vi "AlliGator Image Actions.vi"(0 "AlliGator Q Elements":T6[](array[typedef]), 1 "VI in":refnum<vi>, 2 "Script in":bool, 5 "AlliGator IV DVR in":refnum<data-value>, 7 "AlliGator Q Event in":T7=enum."GUI:Idle", 9 "Data":variant, 11 "error in (no error)":errorcluster, 12 "AlliGator Ctrl Refnums":T8) -> (3 "Script out":bool, 4 "Alligator Queue Elements":T6[](array[typedef]), 6 "AlliGator IV DVR out":refnum<data-value>, 10 "[Notebook Message]":T1[](array[typedef]) {"Message Style"."Font Size" min=6.0 step=1.0}, 15 "error out":errorcluster)   [LabVIEW 2021, in "AlliGator Action Engine.lvlib"]
doc: "Processes AlliGator source image-related actions."
uses:
  AlliGator Action Engine.lvlib
  Internal Variables/AlliGator Internal Variables v2.ctl
  <vilib>/vision/Image Controls.llb/IMAQ Image.ctl
  Internal Variables/AlliGator Gate Image Set.ctl
  Files/AlliGator FLI Dataset Type.ctl
  Files/AlliGator Data Series Type.ctl
  Dual-Channel Datasets/AlliGator Dataset Channel.ctl
  Settings/AlliGator Gate Arithmetic.ctl
  Source Image/AlliGator Displayed Image.ctl
  Image/Named ROI Description.ctl
  Phasor Graph/AlliGator Decay Metadata v3.ctl
  Decay Analysis/Decay Preprocessing/AlliGator Decay Background Subtraction Info.ctl
  Decay Analysis/Decay Preprocessing/AlliGator Baseline Subtraction Method.ctl
  Graphs/XY Graph/XY Graph Plot Shift Parameters.ctl
  Graphs/XY Graph/XY Graph Plot Shift Method.ctl
  Decay Analysis/Decay Preprocessing/AlliGator Decay Extrapolation Parameters.ctl
  Phasor/Calibration Phasor (m, phi).ctl
  Phasor/Phasor Reference Series.ctl
  Phasor/Phasor Calibration Map v2.ctl
  Phasor/Phasor (g, s).ctl
  Phasor Graph/AlliGator Raw Phasor Plot Data v5.ctl
  Phasor/Phasor Standard Deviation Options.ctl
  Phasor Plot/AlliGator Phasor Multi-Harmonic Data.ctl
  Phasor/Phasor Harmonic Data.ctl
  Decay Fit Parameter Map/AlliGator Decay Fit Options & Parameters v4.ctl
  Fits/IRF(X)PSED/Decay Fit Options v4.ctl
  Fits/Decay Convolution/Decay Model.ctl
  Fits/Residual Type.ctl
  Fits/IRF(X)PSED/Fit Weights Type v2.ctl
  Fits/Non-linear Fitting Method v2.ctl
  Fits/Fit Calculation Method.ctl
  Fits/Non-linear Fitting Algorithm.ctl
  Decay Analysis/Decay Fit/AlliGator Decay Fit Parameter Constraints 2.ctl
  Fits/IRF(X)PSED/Decay Fit Parameters In List.ctl
  Fits/IRF(X)PSED/MLE Baseline Offset Type.ctl
  Decay Analysis/Decay Preprocessing/AlliGator Decay Preprocessing Parameters.ctl
  Fits/IRF(X)PSED/Decay Fit Parameters & Derived Quantities List v2.ctl
  Fits/IRF(X)PSED/Decay Fit Result Constraint.ctl
  Decay Fit Parameter Map/AlliGator Parameter Maps Data.ctl
  AlliGator Q Event.ctl
  GUI/AlliGator Ctrl Refnums.ctl
  GUI/AlliGator Other Ctrl Refnums.ctl
  GUI/AlliGator State Indicator.ctl
  GUI/AlliGator Main Window Tabs.ctl
  GUI/AlliGator Phasor Plot Ctrl Refnums.ctl
  GUI/AlliGator Phasor Graph Ctrl Refnums.ctl
  Phasor/Phasor Calibration Type.ctl
  GUI/AlliGator Dataset Ctrl Refnums.ctl
  GUI/AlliGator Registered Events Ctrl Refnums.ctl
  GUI/AlliGator Image Histogram Control Refnums.ctl
  Histograms/Linear Histogram Options.ctl
  Histograms/Histogram Bin Option.ctl
  Histograms/Histogram Bin Position.ctl
  Decay Fit Parameter Map/AlliGator Decay Fit Map Control Refnums.ctl
  Parameter Map/AlliGator Parameter Map Control Refnums.ctl
  AlliGator Q Element.ctl
  Notebook/Notebook Message Object.ctl
  Rich Text Box/Text Formatting.ctl
  Rich Text Box/Text Colors.ctl
  Rich Text Box/Text Style.ctl
  Rich Text Box/Text Alignment.ctl
  Alligator Elements Order in Action Stack.ctl
  Globals, Variables, Constants/AlliGator Variables List.ctl
  Palette/Image Palette Information.ctl
  Image/Image Display Palette Type.ctl
  Rich Text Box/Text Format List.ctl
  Image/Image Display to Clipboard Options.ctl
  Settings/AlliGator Settings List.ctl
  ROIs/AlliGator ROI Manager Actions.ctl
  Image/Image Control ROI Description.ctl
  Image/Image Save File Format.ctl
  Files/AlliGator Saved TIFF Image Type.ctl
  ROIs/AlliGator Selected ROI.ctl
  Image/Image Control Refnum.ctl
  Utilities/Read-Write.ctl
  5e39216f-2ed3-4ea3-88fe-69bdc2580e7f.vi
  Variant/Variant to Data/Variant to [String].vi
  Variant/Variant to Data/Variant to String.vi
  AlliGator Add Single Action to Stack.vi
  Variant/Variant to Data/Variant to Boolean.vi
  Variant/Variant to Data/Variant to DBL.vi
  ROIs/AlliGator Source Image ROI Storage [SGL] v3.vi
  AlliGator Add Action Array to Stack.vi
  Variant/Variant to Data/Variant to I32.vi
  <vilib>/Utility/error.llb/Error Cluster From Error Code.vi
  <vilib>/ErrorRing/Error Ring.xnode
  Image/Image.lvlib
  Variant/Variant to Data/Variant to Data.lvlib
  GUI/GUI.lvlib
  Files/AlliGator Files.lvlib
  Image Profile Window/AlliGator Image Profile Window.lvlib
  Source Image/AlliGator Source Image.lvlib
  Globals, Variables, Constants/AlliGator Globals, Variables & Constants.lvlib
  Palette/Palette.lvlib
  Settings/AlliGator Settings.lvlib
  ROIs/AlliGator ROIs.lvlib
  Notebook/AlliGator Notebook.lvlib
  Internal Variables/AlliGator Internal Variables.lvlib
  Python Plugins API/AlliGator Python Plugins.lvlib
  Phasor Calibration/AlliGator Phasor Calibration.lvlib
  Utilities/Utilities.lvlib
  GUI/AlliGator GUI.lvlib
  Notebook/Notebook.lvlib
  Phasor/Phasor.lvlib
  Decay Analysis/Decay Preprocessing/AlliGator Decay Preprocessing.lvlib
  Graphs/XY Graph/XY Graph Add-Ons.lvlib
  Phasor Graph/AlliGator Phasor Graph.lvlib
  Phasor Plot/AlliGator Phasor Plot.lvlib
  Fits/Fits.lvlib
  Decay Analysis/Decay Fit/AlliGator Decay Fit.lvlib
  Decay Fit Parameter Map/AlliGator Decay Fit Parameter Map.lvlib
  Rich Text Box/Rich Text Box.lvlib
  Dual-Channel Datasets/AlliGator Dual-Channel Datasets.lvlib
  Histograms/Histogram Window.lvlib
  Parameter Map/AlliGator Parameter Map.lvlib
panel:
  # "Drop the content of this VI on AlliGator's diagram\nIn AlliGator, replace the subVI template by a new version"
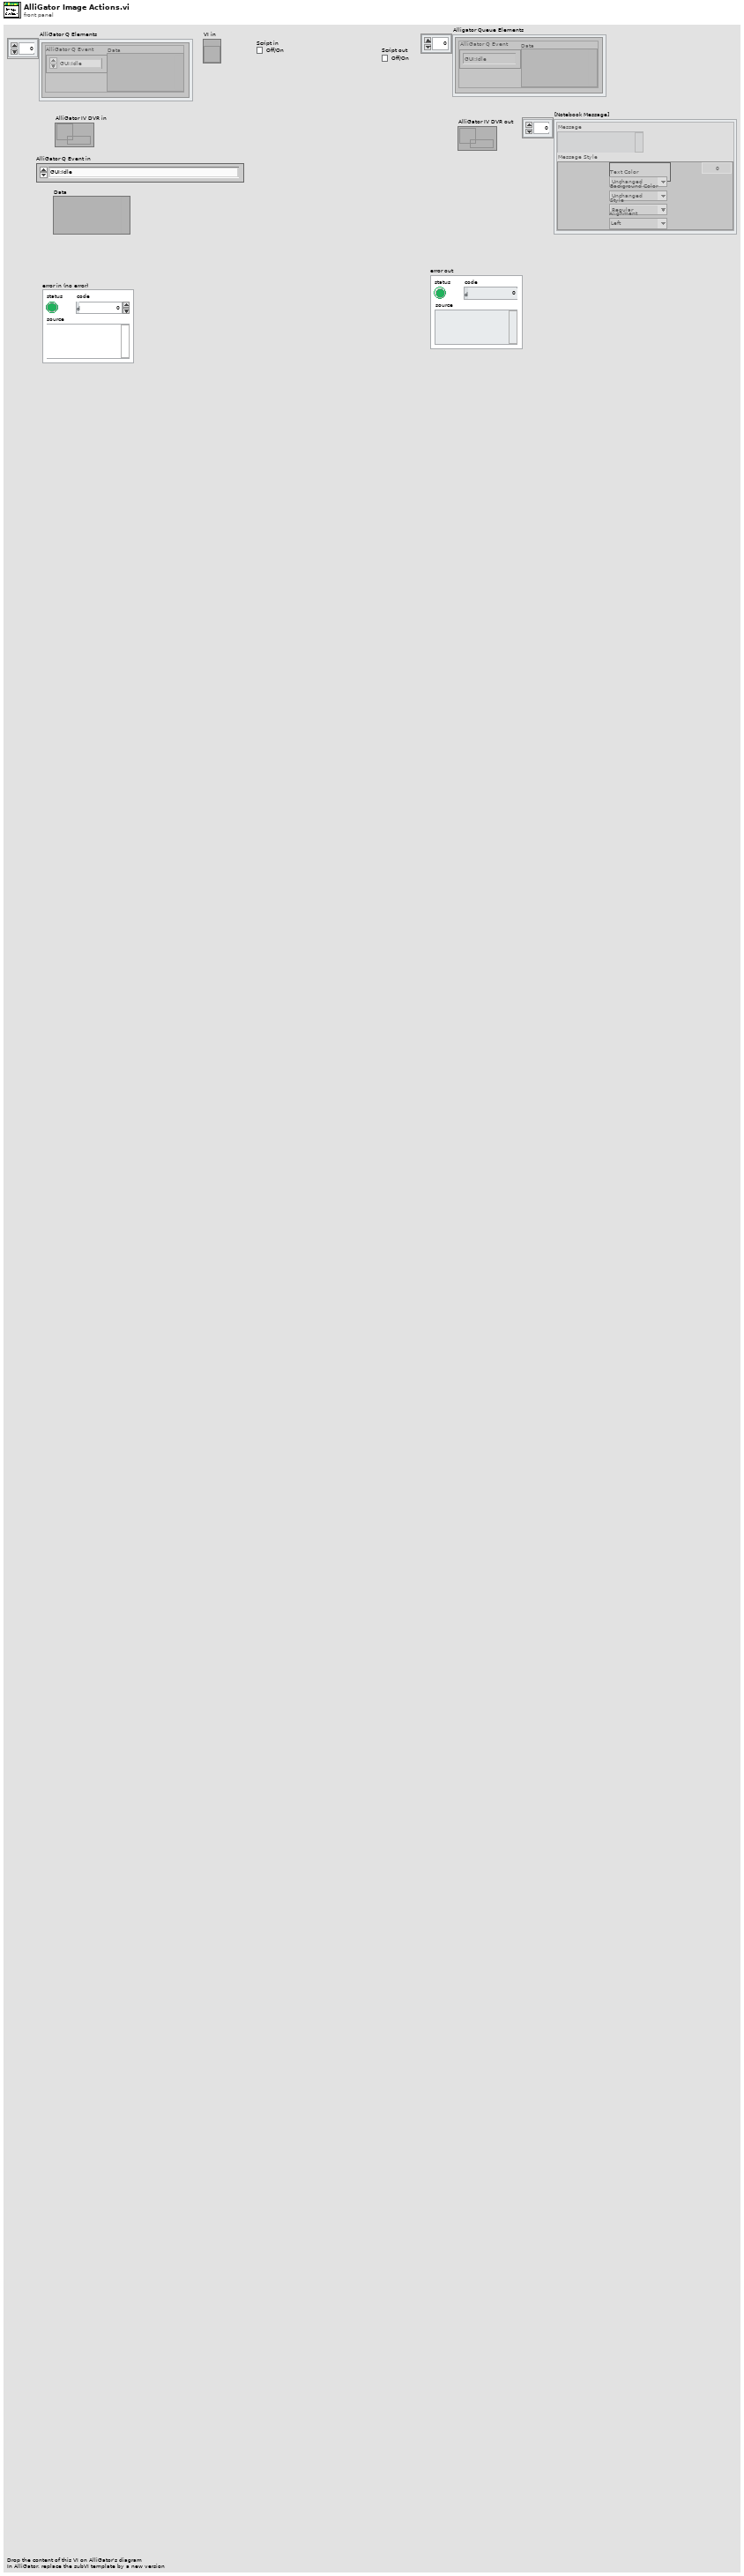
[diagram p1: front panel]
types:
  T1 = typedef "Notebook.lvlib/Notebook Message Object.ctl" = cluster{"Message":string, "Message Style":T2}
  T2 = typedef "Rich Text Box.lvlib/Text Formatting.ctl" = cluster{"Font":string, "Text Color":T3, "Background Color":T3, "Style":T4, "Font Size":dbl, "Alignment":T5}
  T3 = typedef "Rich Text Box.lvlib/Text Colors.ctl" = enum16{"Unchanged", "Black", "Blue", "Cyan", "Maroon", "Gray", "Violet", "Green", "Light Green", "Orange", "Yellow", "Magenta", "Red", "White"}
  T4 = typedef "Rich Text Box.lvlib/Text Style.ctl" = enum16{"Regular", "Bold", "Italic", "Underline", "Strikeout"}
  T5 = typedef "Rich Text Box.lvlib/Text Alignment.ctl" = enum16{"Left", "Right", "Center"}
  T6 = typedef "AlliGator Action Engine.lvlib/AlliGator Q Element.ctl" = cluster{"AlliGator Q Event":T7, "Data":variant}
  T7 = typedef "AlliGator Action Engine.lvlib/AlliGator Q Event.ctl" = enum16{"---- Files ----", "Files:Set Batch Export Files To Save", "Files:Set Dataset Loading & Pre-processing Options", "Files:Check #Frames in Dataset", "Files:Increment Frame Index", "Files:Open Mask Image", "Files:Open White Light Image", "Files:Open Single Dataset", "Files:New Folder of Folders Selected", "Files:Load File (all Types)_Scriptable", "Files:Move Flattened Series to Folders Series", "Files:Select Folder", "Files:Load FLI Dataset", "Files:Load Swiss SPAD 1 Dataset", "Files:Load Swiss SPAD 2 Dataset", "Files:Load .sdt FLI Dataset", "Files:Load .ptu FLI Dataset", "Files:Load .bin FLI Dataset", "Files:Load Single Gate Image Folder", "Files:Load I/m/phi Dataset (deprecated)", "Files:Load Single Image", "Files:Subtract Background File", "Files:Export FLI Dataset", "Files:Load HDF5 FLI Dataset", "Files:Set Destination File Path", "Files:Save Mask Image", "Files:Batch Conversion", "Files:New Folder Selected", "Files:Close FLI Dataset", "Files:Close FLI Dataset Series", "Files:Close White Light Image", "Files:Close Mask Image", "---- FLI Dataset ----", "FLI Dataset:Channel Arithmetic", "FLI Dataset:Export Average Lifetime Map as ASCII", "FLI Dataset:Export User-Defined Quantity Map as ASCII", "FLI Dataset:Python Function FLI Dataset Event", "FLI Dataset:ROI Analysis", "FLI Dataset:Tilted Logistic Square Gated IRF Characteristics Map", "FLI Dataset:Logistic Square Gated IRF Characteristics Map", "FLI Dataset:Square Gated IRF Characteristics Map", "FLI Dataset:Multi-ROI Single-Pixel Phasor Analysis", "FLI Dataset:Multi-ROI Single-Pixel NLSF Analysis", "FLI Dataset:All ROIs IRF Extraction", "FLI Dataset:All ROIs Decay Fit Non-Interactive (Fast + Individual IRF)", "FLI Dataset:All ROIs Phasor Analysis", "FLI Dataset:All ROIs Decay Fit", "FLI Dataset:Fluorescence Decay Statistics", "FLI Dataset:Update Decay Statistics Graph", "FLI Dataset:Get Decay from ROI", "FLI Dataset:All ROIs Average Lifetimes", "FLI Dataset:Save/Load Local IRFs", "FLI Dataset:Clear Local IRFs", "FLI Dataset:Phasor Calibration Maps (# Gates Series) Script", "FLI Dataset:Calibrated Phasor Map Series", "---- FLI Dataset Series ----", "FLI Dataset Series:Sum All Datasets in Series", "FLI Dataset Series:Add Dataset to Accumulated Dataset", "FLI Dataset Series:Display Accumulated Dataset", "FLI Dataset Series:Clear Dataset Series Sum", "FLI Dataset Series:Time-Series Analysis (NLSF)", "FLI Dataset Series:Time-Series Analysis (Phasor)", "---- Image ----", "Image:Update Image Profile Plots", "Image:Image Histogram Cursor Move", "Image:Image Histogram", "Image:Image Contrast", "Image:Set Image Histogram Cursor Move Flag", "Image:Clear Image Overlay", "Image:Use ROI as Search Area", "Image:Set ROI Diameter", "Image:Save Image Data as TIFF", "Image:Save Displayed Image with Overlay", "Image:Save Image Overlay Only", "Image:Save Image as Hot Pixel Mask", "Image:Change Source Image Color Palette", "Image:Copy Image to Clipboard", "Image:Source Image ROI Selection", "Image:Delete All ROIs", "Image:Delete All Unselected ROIs", "Image:Delete ROI", "Image:Merge All ROIs", "Image:Store ROI", "Image:Source Image ROI Storage", "Image:Export ROI Description to Notebook", "Image:Save ROI", "Image:Load ROI", "Image:Paste ROI Definition", "Image:Clear ROI", "Image:Identify ROIs in Mask Image", "Image:Create Complementary ROI", "Image:Create Contour ROI", "Image:Create ROI(s) from Pixels with Peak above Min_Scriptable", "Image:Create ROI(s) from Pixels with Intensity above Min_Scriptable", "Image:Compute ROI Statistics", "Image:Delete ROI(s) based on ROI Characteristics", "Image:Create ROI Grid", "Image:ROI to Individual Pixel ROIs", "Image:Python Function Source Image Event", "Image:Show Phasor Calibration Map ROI Centers", "Image:Convert ROI to Mask Image", "Image:Mouse Move", "Image:Mouse Up", "Image:Set Source Image Mouse Move Flag", "Image:Add Scale Bar Overlay", "Image:Delete Existing ROIs Option", "Image:Overlay ROI Median", "Image:Check Current ROI", "Image:Update True Pixel Value", "---- Decay ----", "Decay:Clear IRF/Reference Plot", "Decay:Add Decay to Graph", "Decay:Smoothen Plot", "Decay:Smoothen Plot Tail", "Decay:Average Selected Plots", "Decay:Extract IRF", "Decay:Optimal IRF Extraction", "Decay:Threshold IRF", "Decay:Fit to Model IRF", "Decay:Fit IRF to Square Gate", "Decay:Fit IRF to Logistic Square Gate", "Decay:Fit IRF to Tilted Logistic Square Gate", "Decay:Create Bounding Cursors Set", "Decay:Export Bounding Cursors Definition to Notebook", "Decay:Denoise Plot", "Decay:Compute Cumulative Function", "Decay:Use as Reference Decay", "Decay:Show Reference Decay/IRF", "Decay:Extrapolate Decay", "Decay:Create Head & Tail Bounding Cursors", "Decay:Store Cursor-defined Head & Tail Fractions", "Decay:Rebin Plot", "Decay:1-Normalize Decay", "Decay:[0-1]-Normalize Plot", "Decay:Straighten Decay", "Decay:Shift Decay", "Decay:Fold Decay", "Decay:Fit Decay", "Decay:Global Fit of Selected Decays", "Decay:Post Global Fit Script", "Decay:Add Global Fit Parameters to Graph", "Decay:Add Decay Parameter(s) to Plot (Graph)", "Decay:Export Decay to Phasor Graph", "Decay:Compute Average Lifetime", "Decay:Plot Convolution", "Decay:Graph Tip Strip Update", "---- Decay Statistics ----", "Decay Statistics:Tip Strip Update", "---- Intensity Time Trace ----", "Intensity Time Trace:Use File Timestamp", "Intensity Time Trace:Load Intensity Corrections File", "Intensity Time Trace:Clear Intensity Corrections File", "Intensity Time Trace:Tip Strip Update", "---- Phasor Plot ----", "Phasor Plot:Build Phasor Plot", "Phasor Plot:Change Phasor Plot Color Palette", "Phasor Plot:Adjust Phasor Plot Display Range", "Phasor Plot:Highlight Image ROI in Phasor Plot", "Phasor Plot:Save Phasor Plot Image with Overlay", "Phasor Plot:Export Complex Phasor Map", "Phasor Plot:Export Phasor Ratio Map", "Phasor Plot:Export Average Lifetime Map", "Phasor Plot:Compute Phase Lifetime Histogram", "Phasor Plot:Compute Phasor Ratio Histogram", "Phasor Plot:Compute Phase Lifetime vs Intensity Scatter Plot", "Phasor Plot:Weber 2-Component Decomposition", "Phasor Plot:Update Phasor Color Map Vertices", "Phasor Plot:Clear Phasor Overlay", "Phasor Plot:Use Segment Extremities as References", "Phasor Plot:Use UC/Segment Intersections as References", "Phasor Plot:Use UC/Principal Axis Intersections as References", "Phasor Plot:Use UC/Linear Fit Intersections as References", "Phasor Plot:Update Phasor Plot Reference", "Phasor Plot:Show Local Phasor Info in Phasor Plot", "Phasor Plot:Update Phasor Plot State", "Phasor Plot:Phasor Plot ROI Storage", "Phasor Plot:Phasor Plot ROI Selection", "Phasor Plot:Python Function Phasor Plot Event", "Phasor Plot:Overlay Phasor ROI, Ratio or Map in Source Image", "Phasor Plot:Compute Decay of Selected Phasors", "Phasor Plot:Phasor at Image Pixel", "Phasor Plot:Mouse Move", "Phasor Plot:Mouse Up", "Phasor Plot:Display Range Mouse Move", "Phasor Plot:Set Mouse Move Flag", "Phasor Plot:Update True Phasor Plot Value", "---- Phasor Graph ----", "Phasor Graph:Get Phasor Value", "Phasor Graph:Create New Phasor Plot Dialog", "Phasor Graph:Update Last Phasor Value", "Phasor Graph:Update Phasor (m, phi)", "Phasor Graph:Remove Single Phasor from Plot", "Phasor Graph:Add Single Phasor to Plot", "Phasor Graph:Remove Phasor Plot", "Phasor Graph:Remove Selected Phasor Plots", "Phasor Graph:Clear Phasor Data", "Phasor Graph:Clear Phasor Graph", "Phasor Graph:Cursor Move", "Phasor Graph:Draw Cursor Connecting Line", "Phasor Graph:Clear Cursor Connecting Line", "Phasor Graph:Find UC Intersection", "Phasor Graph:Use UC/Cursor-Defined Line Intersections", "Phasor Graph:Use Selected Plots Fitted Line/UC Intersections", "Phasor Graph:Use Selected Plots Principal Axis/UC Intersections", "Phasor Graph:Show Single Phasor", "Phasor Graph:Save Single Phasor Plot", "Phasor Graph:Save All Phasor Plots", "Phasor Graph:Load Phasor Plot(s)", "Phasor Graph:Phasor Multiplication", "Phasor Graph:Compute Average Phasor", "Phasor Graph:Compute Multiple Average Phasors (Selected Plots)", "Phasor Graph:Export Single Phasor Plot Phase Lifetimes", "Phasor Graph:Parameter 2 vs Parameter 1 Scatter Plot", "Phasor Graph:Use Cursor n Location", "Phasor Graph:Set Reference n to Current Phase Lifetime Value", "Phasor Graph:Set Reference n to Lifetime Value", "Phasor Graph:Set Cursor n Location", "Phasor Graph:Save Phasor Graph Image", "Phasor Graph:Update SEPL Plot", "Phasor Graph:Export Single Phasor Plot Data", "Phasor Graph:Export Selected Phasor Plots Data", "Phasor Graph:Python Function Phasor Graph Event", "Phasor Graph:Tip Strip Update", "---- Calibration ----", "Calibration:Set Calibration Type", "Calibration:Load/Save Phasor Calibration", "Calibration:Load/Save Phasor Calibration Series", "Calibration:Load/Save Phasor Calibration Map", "Calibration:Use as Calibration", "Calibration:Compute Optimal Calibration from Phasor References", "Calibration:Clear Phasor Calibration", "Calibration:Single Phasor Calibration Information", "Calibration:Use as Calibration Series", "Calibration:Use as Calibration Map", "Calibration:Clear Calibration Series", "Calibration:Phasor Calibration Series Information", "Calibration:Clear Calibration Map", "Calibration:Phasor Calibration Map Information", "Calibration:Apply Phasor Calibration", "Calibration:Update Single Plot Calibration", "Calibration:Update Multiple Plots Calibration", "Calibration:Clear Single Plot Calibration", "Calibration:Clear All Plots Calibrations", "Calibration:Clear Plot(s) Calibration(s)?", "---- Phasor Ratio ----", "Phasor Ratio:Clear Reference n", "Phasor Ratio:Toggle Selected Plot(s)  Lock to Reference 1", "Phasor Ratio:Use as Reference n", "Phasor Ratio:Send Reference n to Notebook", "Phasor Ratio:Toggle Selected Plot(s)  Lock to Reference 2", "Phasor Ratio:Compute Phasor Ratio at Mouse Location", "Phasor Ratio:Compute Phasor Plot's Average Phasor Ratio", "Phasor Ratio:Compute Time-Series Phasor Ratios", "Phasor Ratio:Fit Line to Phasor Ratio Plot", "Phasor Ratio:Save References", "Phasor Ratio:Load References", "Phasor Ratio:Update Phasor Reference 1", "Phasor Ratio:Update Phasor Reference 2", "Phasor Ratio:Move Cursor n to Reference n", "Phasor Ratio:Use as Phasor Reference 1 Lifetime", "Phasor Ratio:Use as Phasor Reference 2 Lifetime", "Phasor Ratio:Export Phasor Ratio Map as ASCII", "Phasor Ratio:Tip Strip Update", "---- Lifetime & Other Parameters Graph ----", "Lifetime:Compute Sliced Mean, SDV and CV Plots", "Lifetime:Plot Decay Shifts", "Lifetime:Plot Histogram", "---- Decay Fit Parameter Map ----", "Decay Fit Parameter Map:Export ROI NLSF Data as ASCII", "Decay Fit Parameter Map:Set Decay Fit Parameter Map Selection", "Decay Fit Parameter Map:Build Decay Fit Parameter Map", "Decay Fit Parameter Map:Change Decay Fit Parameter Map Color Palette", "Decay Fit Parameter Map:Export Decay Fit Parameter Map Data as ASCII", "Decay Fit Parameter Map:Export All Decay Fit Parameter Maps Data as ASCII", "Decay Fit Parameter Map:Selected Parameter Scatterplot", "Decay Fit Parameter Map:Parameter 2 vs Parameter 1 Scatterplot", "Decay Fit Parameter Map:Save Decay Fit Parameter Map Image", "Decay Fit Parameter Map:Save-Load IRFs & Fit Data", "Decay Fit Parameter Map:Update Local Decay Plots", "Decay Fit Parameter Map:Python Function Decay Fit Parameters Map Event", "Decay Fit Parameter Map:Overlay Decay Fit Parameter Map in Source Image", "Decay Fit Parameter Map:Selected Parameter vs Intensity Scatterplot", "Decay Fit Parameter Map:Mouse Up", "Decay Fit Parameter Map:Mouse Move", "Decay Fit Parameter Map:Display Range Mouse Move", "Decay Fit Parameter Map:Change Map Resolution", "Decay Fit Parameter Map:Variance Significance Maps", "Decay Fit Parameter Map:Fit Result Constraints Window", "---- Parameter Map ----", "Parameter Map:Export ROI Parameters Data as ASCII", "Parameter Map:Add Parameter Map Set", "Parameter Map:Delete Parameter Map Set", "Parameter Map:Update Parameter List", "Parameter Map:Build Parameter Map", "Parameter Map:Change Parameter Map Color Palette", "Parameter Map:Export Parameter Map Data as ASCII", "Parameter Map:Export All Parameter Maps Data as ASCII", "Parameter Map:Selected Parameter Scatterplot", "Parameter Map:Parameter 2 vs Parameter 1 Scatterplot", "Parameter Map:Selected Parameter vs Intensity Scatterplot", "Parameter Map:Save Parameter Map Image", "Parameter Map:Save-Load IRFs & Parameter Maps (TODO)", "Parameter Map:Set Parameter Map Selection", "Parameter Map:Python Function Parameter Map Event", "Parameter Map:Overlay Parameter Map in Source Image", "Parameter Map:Update Local Decay Plots", "Parameter Map:Mouse Up", "Parameter Map:Mouse Move", "Parameter Map:Display Range Mouse Move", "---- Generic Graph ----", "Generic Graph:Generic XY Graph Event", "Generic Graph:Python Function XY Graph Event", "Generic Graph:New Plot", "Generic Graph:Save Plot", "Generic Graph:XY Plot Histogram", "Generic Graph:Set XY Graph Plot Name", "Generic Graph:Set Last Cursor Style", "Generic Graph:Tip Strip Update", "---- GUI ----", "GUI:Start Script", "GUI:Type of Displayed Image Changed", "GUI:Gate Image Slide Changed", "GUI:Show Busy Icon", "GUI:Show Busy Icon & Abort Button", "GUI:Hide Busy Icon", "GUI:Hide Busy Icon & Abort Button", "GUI:Abort", "GUI:End Script", "GUI:Start Timing", "GUI:End Timing", "GUI:Set State Indicator", "GUI:Send Parameters JSON Strings to Clipboard", "GUI:Set Gate Step", "GUI:Idle", "GUI:Initialization", "GUI:Quit", "GUI:Increment Dataset Index", "GUI:Set Dataset Index to -1", "GUI:Time Series Slider Moved", "GUI:Time Series Slider Changed", "GUI:Toggle Playback or Loop", "GUI:Playback Script", "GUI:Set Phasor Frequency", "GUI:Open Window", "GUI:Start Test Script", "GUI:End Test Script", "GUI:Set Verbose Mode", "GUI:Set Verbose Settings Mode", "DEBUG"}
  T8 = typedef "AlliGator GUI.lvlib/AlliGator Ctrl Refnums.ctl" = cluster{"Other AlliGator Ctrl Refnums":T9, "Phasor Plot Ctrl Refnums":T10, "Phasor Graph Ctrl Refnums":T11, "Dataset Control Refnums":T12, "Registered Events Ctrl Refnums":T13, "Image Histogram Ctrl Refnums":T14, "Decay Fit Map Ctrl Refnums":T15, "Parameter Map Ctrl Refnums":T16}
  T9 = typedef "AlliGator GUI.lvlib/AlliGator Other Ctrl Refnums.ctl" = cluster{"State Indicators":refnum<vi>, " Progress Bar":refnum<vi>, "Decay Graph Active":refnum<vi>, "Decay Statistics Bin":refnum<vi>, "Time Step":refnum<vi>, "Use File Timestamp":refnum<vi>, "Tab Control":refnum<vi>, "CPU":refnum<vi>, "Abort Fit":refnum<vi>, "Dataset File/Folder Path":refnum<vi>, "Abort ROI Creation":refnum<vi>, "Event LED":refnum<vi>, "Dataset File/Folder Path 2":refnum<vi>, "Dataset File/Folder Path 3":refnum<vi>, "Dataset File/Folder Path 4":refnum<vi>, "Dataset File/Folder Path 5":refnum<vi>, "Dataset File/Folder Path 6":refnum<vi>, "Dataset File/Folder Path 7":refnum<vi>, "Dataset File/Folder Path 8":refnum<vi>, "Dataset File/Folder Path 9":refnum<vi>, "Dataset File/Folder Path 10":refnum<vi>, "Dataset File/Folder Path 11":refnum<vi>}
  T10 = typedef "AlliGator GUI.lvlib/AlliGator Phasor Plot Ctrl Refnums.ctl" = cluster{"Phasor Ratio":refnum<vi>, "Modulus Lifetime":refnum<vi>, "Phasor at cursor (m, phi)":refnum<vi>, "Phase Lifetime":refnum<vi>, "Phasor at cursor (g, s)":refnum<vi>, "Phasor Plor Average Lifetime":refnum<vi>, "Phasor Plot Active":refnum<vi>, "Save Phasor Plot":refnum<vi>, "Image Overlay Color":refnum<vi>, "Phasor Plot Color Scale":refnum<vi>, "Reference 1 Button":refnum<vi>, "Reference 2 Button":refnum<vi>, "True Phasor Plot Value":refnum<vi>}
  T11 = typedef "AlliGator GUI.lvlib/AlliGator Phasor Graph Ctrl Refnums.ctl" = cluster{"Phasor Ratio":refnum<vi>, "Modulus Lifetime":refnum<vi>, "Phasor at cursor (m, phi)":refnum<vi>, "Phase Lifetime":refnum<vi>, "Phasor at cursor (g, s)":refnum<vi>, "Phasor Graph Average Lifetime":refnum<vi>, "Phasor Graph Active":refnum<vi>, "Save Phasor Graph":refnum<vi>, "Phasor Frame Slide":refnum<vi>, "Single Step Phasor":refnum<vi>, "Calibration Type":refnum<vi>, "Show Line":refnum<vi>, "Phase Lifetime 1":refnum<vi>, "Phase Lifetime 2":refnum<vi>, "Phasor Graph Frequency":refnum<vi>, "Phasor Reference 1 Control":refnum<vi>, "Phasor Reference 2 Control":refnum<vi>, "Calibration Lifetime":refnum<vi>, "Phase Lifetime SDV":refnum<vi>, "Average Lifetime SDV":refnum<vi>, "Phasor Ratio SDV":refnum<vi>, "Modulus Lifetime SDV":refnum<vi>}
  T12 = typedef "AlliGator GUI.lvlib/AlliGator Dataset Ctrl Refnums.ctl" = cluster{"Current Data":refnum<vi>, "Gate Image Slide":refnum<vi>, "Time Point Slide":refnum<vi>, "Current Time Stamp":refnum<vi>, "Save Image":refnum<vi>, "Displayed Image":refnum<vi>, "Overlay Mode":refnum<vi>, "Phasor Overlay Color":refnum<vi>, "Image Color Scale":refnum<vi>, "Use ROI as Search Area":refnum<vi>, "Source Image ROI Color":refnum<vi>, "True Pixel Value":refnum<vi>}
  T13 = typedef "AlliGator GUI.lvlib/AlliGator Registered Events Ctrl Refnums.ctl" = cluster{"Time Point Slider":refnum<vi>, "Phasor Plot Display Range":refnum<vi>, "Decay Graph":refnum<vi>, "Decay Statistics Graph":refnum<vi>, "Intensity Time Trace":refnum<vi>, "Phasor Graph":refnum<vi>, "Phasor Ratio Graph":refnum<vi>, "Lifetime Graph":refnum<vi>, "Phasor Plot Display":refnum<vi>, "Source Image Display":refnum<vi>, "Decay Fit Parameter Map Display Range":refnum<vi>, "Decay Fit Parameter Map Display":refnum<vi>, "Parameter Map Display Range":refnum<vi>, "Parameter Map Display":refnum<vi>, "Phasor Plot Display Range":refnum<vi>}
  T14 = typedef "AlliGator GUI.lvlib/AlliGator Image Histogram Control Refnums.ctl" = cluster{"Image Histogram":refnum<vi>, "Image Histogram Options":refnum<vi>, "Image Histogram Active":refnum<vi>, "Image Histogram Upper Percentile":refnum<vi>, "Image Histogram Lower Percentile":refnum<vi>, "Auto-Adjust Contrast":refnum<vi>}
  T15 = typedef "AlliGator Decay Fit Parameter Map.lvlib/AlliGator Decay Fit Map Control Refnums.ctl" = cluster{"Decay Fit Parameter Map Color Scale":refnum<vi>, "Decay Fit Parameter":refnum<vi>, "Max Parameter":refnum<vi>, "Min Parameter":refnum<vi>, "Decay Fit Parameter Map Display":refnum<vi>, "Decay Fit Parameter Map Display Range":refnum<vi>, "Decay Parameter Map X":refnum<vi>, "Decay Parameter Map Y":refnum<vi>, "Decay Parameter Map Value":refnum<vi>}
  T16 = typedef "AlliGator Parameter Map.lvlib/AlliGator Parameter Map Control Refnums.ctl" = cluster{"Parameter Map Color Scale":refnum<vi>, "Map Parameter":refnum<vi>, "Max Parameter":refnum<vi>, "Min Parameter":refnum<vi>, "Parameter Map Display":refnum<vi>, "Parameter Map Display Range":refnum<vi>, "Parameter Map Set":refnum<vi>, "Parameter Map X":refnum<vi>, "Parameter Map Y":refnum<vi>, "Parameter Map Value":refnum<vi>}
  T17 = typedef "AlliGator Action Engine.lvlib/Alligator Elements Order in Action Stack.ctl" = enum16{"Enqueue 2 AFTER 1", "Enqueue 2 BEFORE 1"}
  T18 = typedef "AlliGator Globals, Variables & Constants.lvlib/AlliGator Variables List.ctl" = enum16{"---- GUI ----", "GUI:Initialization Status", "GUI:State Indicators Refnum", "GUI:Original AlliGator Menu Items", "GUI:Current Action Loop State", "GUI:Script in progress", "GUI:Playback", "GUI:Loop Playback", "GUI:Search ROI Used", "GUI:Search ROI", "Decay Graph Max Legend Size", "Intensity Graph Max Legend Size", "Decay Statistics Graph Max Legend Size", "Phasor Graph Max Legend Size", "Phasor Ratio Graph Max Legend Size", "Lifetime Graph Max Legend Size", "---- Files ----", "Files:Export Dataset Frames as Individual Files", "Files:Show Batch Export Help Balloons", "Files:Frames in Dataset", "Files:ptu File Frame Start Indices", "Files:Current Frame in Dataset", "Files:Current Frame Timestamp", "Files:Dataset Loaded", "Files:Dataset Metadata", "Files:Dataset Channel", "Files:Dataset Data Description", "Files:Background Dataset Metadata", "Files:Background Dataset Channel", "Files:Background Dataset Data Description", "Files:Background File Subtraction", "Files:Background File Path", "Files:Background File Pile-up Correction", "Files:Background File Pixel Well Capacity", "Files:Background File Scaling Factor", "Files:Current Dataset Load Settings", "Files:Dataset Path", "Files:ICCD-specific Information", "Files:Macrotime Gate Separation", "------ Python Plugins ------", "Python Plugins:Information", "Python Plugins:Python Session", "Python Plugins:Valid Python Session?", "---- Source Image ----", "Source Image:ROIs", "Source Image:Current ROI", "Source Image:ROI Event Refnum", "X_Source Image:Display Range", "X_Source Image:Palette Information", "X_Source Image:Type of Displayed Image", "X_Time Gate Slider", "Source Image:Palette List", "Source Image:Scale", "Source Image:ROI Overlay Color", "Source Image:Overlay to Erase", "Source Image:Is Displayed Image Accumulated", "Source Image:White Light Image Modified", "Source Image:Mask Image Modified", "---- Image Profile Window ----", "Image Profile:Window Event Refnum", "Image Profile:IntensityType", "Image Profile:Intensity Average Type", "Image Profile:Intensity-weighted SDV", "Image Profile:Box Profile Type", "Image Profile:Window Open", "Image Profile:Plotted Fit Parameter", "------ Phasor Graph -------", "Phasor Graph:Show Line", "---- Phasor Plot ---", "Phasor Plot:Parameters Changed", "Phasor Plot:FLI Dataset Modified since last Calculation", "Phasor Harmonics Data", "Selected Phasor Harmonics", "Phasor Harmonic Manager Event Refnum", "Phasor Plot:ROIs", "Phasor Plot:Current ROI", "Phasor Plot:ROI Event Refnum", "Phasor Plot:Image Reference Points", "Phasor Plot:Computed", "Phasor Plot:Palette Information", "Phasor Plot:Palette List", "Phasor Plot:Phasor Ratio Palette Information", "Phasor Plot:Phasor Ratio Palette List", "Phasor Plot:Image Scale", "Phasor Plot:Image Overlay to Erase", "Phasor Plot:Image Elements to Update", "Phasor Plot:Current Calculation Parameters", "Phasor Plot:Current Calibration Options", "Phasor Plot:Reset Cumulated Phasor Plot", "Phasor Plot:Reference 1", "Phasor Plot:Lifetime Reference 1", "Phasor Plot:Reference 1 Frequency", "Phasor Plot:Reference 2", "Phasor Plot:Lifetime Reference 2", "Phasor Plot:Reference 2 Frequency", "---- Decay Analysis ----", "Number of Selected Decays to Fit", "LS Fit Results", "LAR Fit Results", "BS Fit Results", "Last Decay Max - Min", "Best Fit Parameters", "Best Fit Parameter Names", "Actual Size X", "Actual Size Y", "Binning X", "Binning Y", "Actual # Gates", "Dataset Number", "Gates to...", "Gates Skipped", "Gates to keep", "Gate Step", "Gate Separation", "Reversed Gates", "Pile-up Correction", "Pixel Well Capacity", "Background Subtracted", "Background Subtraction Method", "Background Definition Range", "Background File (deprecated)", "Number of Dataset Accumulated", "Array of Accumulated Dataset Paths", "Do Averaged Datasets", "Destination File Path", "Process Plot Target", "Use 1/D as Phasor Frequency", "---- Decay Fit Parameter Map -----", "Decay Fit Parameter Map:Palette Information", "Decay Fit Parameter Map:Palette List", "Decay Fit Parameter Map:X Resolution", "Decay Fit Parameter Map:Y Resolution", "Decay Fit Parameter Map:Use Decay Fit Result Constraints", "Decay Fit Parameter Map:Decay Fit Result Constraints", "Decay Fit Parameter Map:Decay Fit Result Constraints Applied", "---- Parameter Map ----", "Parameter Map:Palette Information", "Parameter Map:Palette List", "------- Local Decay Window ---------", "Local Decay Graph Window:Event Refnum", "Local Decay Graph Window:Use normalized IRF for convolution", "----- Miscellaneous ----", "Misc:Skippable Dialog Windows Status"}
  T19 = typedef "Palette.lvlib/Image Palette Information.ctl" = cluster{"Palette Name [# Colors,int?,inv?]":string, "Palette Type":T20, "Palette Colors":u32[], "Interpolate?":bool}
  T20 = typedef "Image.lvlib/Image Display Palette Type.ctl" = u32
  T21 = typedef "Notebook.lvlib/Text Format List.ctl" = enum16{"Message", "Result", "Error", "Setting", "Verbose", "Warning"}
  T22 = typedef "Image.lvlib/Image Display to Clipboard Options.ctl" = cluster{"Include Overlay (T)":bool, "Image Only (T)":bool}
  T23 = cluster{"CtlRef":refnum<vi>, "Image to Clipboard Options":T22}
  T24 = typedef "AlliGator Settings.lvlib/AlliGator Settings List.ctl" = enum16{"GUI:Visible Settings Tab", "GUI:Last Run Version", "Source Image:Use Image Histogram for Contrast", "Source Image:Low Count Pixels Rejection Options", "Source Image:High Count Pixels Rejection Options", "Source Image:Use Image Brightness", "Source Image:Blend Overlay with Image Background", "Source Image:Use Fixed ROI Diameter", "Source Image:ROI Diameter", "Source Image:ROI Center Color", "Source Image:Peak Threshold", "Source Image:Intensity Threshold", "Source Image:Image Binning Options", "Source Image:Image Smoothing Options", "Source Image:Image Histogram Active", "Source Image:Invert Binary Mask", "Source Image:Hot Pixel Removal", "Source Image:Overlay Analyzed ROI Center", "Source Image:Auto-Adjust Contrast", "Source Image:Histogram Lower Percentile", "Source Image:Histogram Upper Percentile", "Source Image:Save Source Image", "Source Image:Scale Bar Options", "Source Image:Image Resolution (Pixel Size)", "Source Image:Flatfield Correction", "Source Image:Show Dead Left Columns Correction", "Source Image:Dead Left Columns Correction", "Source Image:Image Pre-Processing Operations Order", "Source Image:Overlay ROI Median", "Source Image:Median Overlay Color", "Data Information:Gate Width", "Data Information:Nanotime Gate Separation", "Data Information:Macrotime Gate Separation", "Data Information:Gate Step", "Data Information:# Gates", "Data Information:Gate Image Exposure", "Data Information:Gate Image Integration", "Data Information:Gates to Skip", "Data Information:Gates to Keep", "Data Information:Define Gates to", "Data Information:Channel Name", "Data Information:Available Channel Names", "Data Information:Channel Arithmetic", "Data Information:Background File Subtraction", "Data Information:Background File", "Data Information:Background Scaling Factor", "Data Information:Background Pile-up Correction", "Data Information:Background Pixel Well Capacity", "Data Information:Laser Period", "Data Information:SYNC Period", "Data Information:Pile-up Correction", "Data Information:Pixel Well Capacity", "Data Information:Dataset Scaling Factor", "Fluorescence Decay_Decay Pre-Processing:Reverse Gates", "Fluorescence Decay_Decay Pre-Processing:Verbose Decay Pre-Processing", "Fluorescence Decay_Decay Pre-Processing:Use Decay Pre-Processing", "Fluorescence Decay_Decay Pre-Processing:Background Subtraction", "Fluorescence Decay_Decay Pre-Processing:Background Definition Range", "Fluorescence Decay_Decay Pre-Processing:Baseline Subtraction Method", "Fluorescence Decay_Decay Pre-Processing:Decay Pre-Processing Operations Order", "Fluorescence Decay_Decay Pre-Processing:Smoothing Parameter", "Fluorescence Decay_Decay Pre-Processing:Shift Decay", "Fluorescence Decay_Decay Pre-Processing:Decay Shift Parameters", "Fluorescence Decay_Decay Pre-Processing:Fold Decay", "Fluorescence Decay_Decay Pre-Processing:# Folds", "Fluorescence Decay_Decay Pre-Processing:1-Normalize Decay", "Fluorescence Decay_Decay Pre-Processing:[0-1]-Normalize Decay", "Fluorescence Decay_Decay Pre-Processing:Smoothen Decay", "Fluorescence Decay_Decay Pre-Processing:Extrapolate Decay", "Fluorescence Decay_Decay Pre-Processing:Use Periodicity", "Fluorescence Decay_Decay Pre-Processing:Use Cursors", "Fluorescence Decay_Decay Pre-Processing:Tail Fraction", "Fluorescence Decay_Decay Pre-Processing:Head Fraction", "Fluorescence Decay_Decay Pre-Processing:Additional Points", "Fluorescence Decay_Decay Pre-Processing:Straighten Decay", "Fluorescence Decay_Decay Pre-Processing:Constant Background", "Fluorescence Decay_Decay Pre-Processing:Pixel-Normalize Decay", "Fluorescence Decay_Advanced Analysis:Extract IRF instead of Decay", "Fluorescence Decay_Advanced Analysis:IRF Extraction Options", "Fluorescence Decay_Advanced Analysis:IRF Optimization Options", "Fluorescence Decay_Advanced Analysis:Square Pulse Options", "Fluorescence Decay_Advanced Analysis:IRF Order", "Fluorescence Decay_Advanced Analysis:IRF Time Constants", "Fluorescence Decay_Advanced Analysis:Wavelet Analysis Options", "Fluorescence Decay_Advanced Analysis:Average Lifetime Options", "Fluorescence Decay_Fit Options:Fit Options", "Fluorescence Decay_Fit Options:Use Legacy Fitting Approach", "Fluorescence Decay_Fit Options:Use Data Information Laser Period", "Fluorescence Decay_Fit Parameters:Displayed Fit Parameters", "Fluorescence Decay_Fit Parameters:Fit Parameter Constraints", "Fluorescence Decay_Fit Parameters:Export Tabulated Results", "Fluorescence Decay_Fit Parameters:MLE Baseline Offset Type", "Fluorescence Decay_Fit Parameters:MLE Baseline Offset", "Fluorescence Decay_Fit Parameters:Guess Parameter Names", "Fluorescence Decay_Fit Parameters:Guess Parameter Values", "Fluorescence Decay_Fit Parameters:Guess Parameters Options", "Fluorescence Decay_Fit Parameters:Optimal Offset Selection Criterion", "Fluorescence Decay_Styles:Show Last Decay Only", "Fluorescence Decay_Styles:Decay Graph Color Array", "Fluorescence Decay:Decay Graph Active", "Fluorescence Decay Statistics:Min Peak Value", "Fluorescence Decay Statistics:Reject Low Decay Peak Pixels", "Fluorescence Decay Statistics:Reject High Decay Peak Pixels", "Fluorescence Decay Statistics:Max Peak Value", "Time Traces:Use File Timestamp", "Time Traces:Time Step", "Time Traces:Use Intensity Correction File", "Time Traces:Intensity Correction File", "Phasor Plot:Phasor Plot Smoothing Options", "Phasor Plot:Phasor Plot Size", "Phasor Plot:Phasor Plot Graphics Options", "Phasor Plot:Cumulative Phasor Plot", "Phasor Plot:Use Phasor Brightness", "Phasor Plot:Blend Overlay with Phasor Background", "Phasor Plot:Save Phasor Plot", "Phasor Plot:Show References", "Phasor Plot:Phasor Ratio Decay Range", "Phasor Plot:Exponential Fading", "Phasor Plot:Phasor Ratio Reference Colors", "Phasor Plot:Reference Radius", "Phasor Plot:Show Color Map Vertices", "Phasor Plot:Phasor Plot Active", "Phasor Plot:Phasor Ratio Color Map Type", "Phasor Plot:Phasor Ratio Color Map", "Phasor Plot:Phasor Ratio Display Range", "Phasor Plot:Selected Image ROI(s)", "Phasor Plot:All Image ROIs", "Phasor Plot:Selected Phasor Plot ROI(s)", "Phasor Plot:All Phasor Plot ROIs", "Phasor Plot:Phasor Ratio Color-Coded Quantity", "Phasor Plot:Store Phasor Harmonics", "Phasor Plot:Draw Reference Segment", "Phasor Plot:User-Defined Quantity", "Phasor Plot:Color Scale High Color", "Phasor Plot:Color Scale Low Color", "Phasor Plot:Intensity-weighted Phasor Plot", "Phasor Graph:Phasor Frequency", "Phasor Graph:Phasor Ratio Type", "Phasor Graph:Pixel-level Phasor Computation", "Phasor Graph:Save Phasor Graph", "Phasor Graph:Phasor Graph Active", "Phasor Graph:Phasor SDV Options", "Phasor Graph:Intensity-weighted Phasor Graph", "Phasor Graph:Define Shortest Lifetime as", "Phasor Calibration:Use Backup Calibration if needed", "Phasor Calibration:Backup Calibration Type", "Phasor Calibration:Calibration Type", "Phasor Calibration:Calibration Lifetime", "Phasor Calibration:Calibration Map Algorithm", "Single-Exponential Phasor Locus (SEPL):Gate Parameters", "Single-Exponential Phasor Locus (SEPL):User-defined Gate", "Single-Exponential Phasor Locus (SEPL):User-defined IRF", "Single-Exponential Phasor Locus (SEPL):Phasor Parameters", "Single-Exponential Phasor Locus (SEPL):Decay & IRF Parameters", "Single-Exponential Phasor Locus (SEPL):Display Parameters", "Lifetime Analysis:Decay Analysis Parameters", "Lifetime Analysis:Lifetime Map Active", "Plugins:Python Settings", "Miscellaneous:Verbose Mode", "Miscellaneous:Beep after Script", "Miscellaneous:Saved Image File Format", "Miscellaneous:Exported Gate Image Settings", "Miscellaneous:Include Loading in Timing", "Miscellaneous:Verbose Settings Mode", "Miscellaneous:Histogram Options", "Miscellaneous:Beep on Error", "Miscellaneous:# Logical Processors Used", "Miscellaneous:ROI Description Max Characters", "Miscellaneous:Verbose Error Mode", "Miscellaneous:Transparent Mask Color"}
  T25 = typedef "AlliGator ROIs.lvlib/AlliGator ROI Manager Actions.ctl" = enum16{"Undefined", "Delete Current ROI", "Delete All Unselected ROIs", "Delete Multiple ROIs", "Delete All ROIs", "Swap ROIs", "Insert ROI", "Update Current ROI Descriptor", "Rename Current ROI", "Store New ROI", "Store Multiple ROIs", "Select Next ROI", "Select Previous ROI", "Find Selected ROI", "Show All ROIs", "Update ROI Manager Window", "Merge All ROIs", "Unmerge ROI", "Set Selected ROI by ID"}
  T26 = typedef "ROI Descriptor" = cluster{"Global Rectangle":i32[], "Contours":cluster{"ID":enum32{"External", "Internal"}, "Type":u32, "Coordinates":i32[]}[]}
  T27 = typedef "Image.lvlib/Image Control ROI Description.ctl" = cluster{"Image Control Label":string, "ROI Descriptor":T26}
  T28 = typedef "IMAQ Image.ctl" = refnum<image>
  T29 = typedef "Image.lvlib/Image Save File Format.ctl" = enum16{"PNG", "JPEG", "BMP"}
  T30 = typedef "AlliGator Files.lvlib/AlliGator Saved TIFF Image Type.ctl" = enum16{"Single Gate", "Sum of All Gates", "Phasor"}
  T31 = typedef "AlliGator ROIs.lvlib/AlliGator Selected ROI.ctl" = cluster{"Image Ctrl Ref":T32, "All ROIs?":bool}
  T32 = typedef "Image.lvlib/Image Control Refnum.ctl" = refnum<vi>
  T33 = typedef "Utilities.lvlib/Read-Write.ctl" = enum16{"Read", "Write"}
  T34 = typedef "AlliGator Internal Variables.lvlib/AlliGator Internal Variables v2.ctl" = cluster{"----------------------------- Images -----------------------------":u8, "Displayed Image":T28, "White Light Image":T28, "Mask Image":T28, "ROI Mask Image":T28, "Current Dataset Images 1":T35, "Background Dataset Images 1":T35, "Current Dataset Images 2":T35, "Background Dataset Images 2":T35, "Current Dataset Arithmetic Images":T35, "Accumulated Dataset Images 1":T35, "Accumulated Dataset Images 2":T35, "Accumulated Dataset Arithmetic Images":T35, "----------------------------- File Paths -----------------------------":u8, "Phasor Plot Image":T28, "Decay Fit Parameter Map Image":T28, "Parameter Map Image":T28, "Single Data Point Path":path, "White Light Image Path":path, "Mask Image Path":path, "Time-Series Folder":path, "[Time-Series Paths]":path[], "----------------------------- FLI Dataset -----------------------------":u8, "Current Dataset":i32, "Single Dataset Type":T36, "Current Folder":string, "AlliGator Data Series Type":T37, "# Datasets":i32, "Dual-Channel Dataset":bool, "Selected Channel Name":string, "Dataset Channel":T38, "Channel Arithmetic":T39, "Dual-Channel Background Dataset":bool, "Background Channel":T38, "Dual-Channel Accumulated Dataset":bool, "Start Time":dbl, "[Time-Series Timestamps]":dbl[], "[Intensity Corrections]":dbl[], "Time Series Script":bool, "Type of Displayed Image":T40, "Gate Image Slide":u16, "# Gates":i32, "ROIs":T41[], "----------------------------- Decays -----------------------------":u8, "ROI Decay":cluster{"t Array":dbl[], "I Array":dbl[]}, "Valid Decay":bool, "Decay  Metadata":T42, "Reference Decay Plot Name":string, "Reference Decay":cluster{"t Array":dbl[], "I Array":dbl[]}, "Decay Shift Plot":cluster{"Time Stamps":dbl[], "Decay Shifts":dbl[]}, "[Decays Max Values]":sgl[], "[Decays Min Values]":sgl[], "----------------------------- Calibration -----------------------------":u8, "Calibration Phasor":T48, "Calibration Phasor Series":T49, "Phasor Calibration Map":T50, "Calibration Map MD5 Digest":string, "----------------------------- Phasor Graph -----------------------------":u8, "Last Raw Phasor":T51, "Last Calibrated Phasor":T51, "Last Calibrated Phasor SDV":T51, "Phasor Graph:Phasor Plot":cluster{"g Array":dbl[], "s Array":dbl[]}, "Phasor Graph:Phasor SDV Plot":cluster{"g Array":dbl[], "s Array":dbl[]}, "[Phasor Graph:Raw Phasor Plots]":T52[], "Phasor Plot locked to Ref 1":i32, "[Phasor Plot(s) locked to Ref 1]":i32[], "[Phasor Plot(s) locked to Ref 2]":i32[], "[Pixel Phasors]":T51[], "----------------------------- Phasor Plot -----------------------------":u8, "[[Sum Image]]":dbl[][], "[[CSG Phasors]]":csg[][], "[[Valid Pixel?]]":bool[][], "[[Phasor Ratios]]":dbl[][], "[[Average Lifetimes]]":dbl[][], "Amplitude Weighted Average Lifetime":bool, "I/m/phi Dataset":cluster{"I/m/phi Dataset?":bool, "Base Frequency":dbl[unit], "Harmonic Orders":u8[]}, "Multi Phasor Plot Data":T54, "----------------------------- Decay Fit Parameter Map -----------------------------":u8, "Decay Fit Options & Parameters":T56, "Fit Options: Decay Preprocessing Parameters":T67, "Fit Options: Reference Decay":cluster{"t Array":dbl[], "I Array":dbl[]}, "Is Full Image Parameters Map":bool, "Is Single-Pixels Parameters Map":bool, "NLSF Parameters Map X Resolution":i32, "NLSF Parameters Map Y Resolution":i32, "[Single Decay Fit Parameters]":dbl[], "Fit Model":T58, "[[Multiple Decays Fit Parameters]]":dbl[][], "[[Multiple Decays Fit Parameter SDVs]]":dbl[][], "[[IRFs]]":dbl[][], "[ROI Descriptors]":T26[], "IRF Array Time Axis":dbl[], "Decay Array Time Axis":dbl[], "[Decay Fit Parameter Names]":T68[], "[Decay Sum]":dbl[], "Array of Decay Fit Result Constraints":T69[], "Selected ROIs Array":bool[], "----------------------------- Parameter Maps -----------------------------":u8, "[Map Set Names]":string[], "[Parameter Maps]":T70[], "[[User-defined Quantities]]":dbl[][], "User-defined Quantity":string}
  T35 = typedef "AlliGator Internal Variables.lvlib/AlliGator Gate Image Set.ctl" = cluster{"SGL Gate Images":T28[], "SGL Sum Image":T28, "SGL Max Image":T28, "SGL Min Image":T28}
  T36 = typedef "AlliGator Files.lvlib/AlliGator FLI Dataset Type.ctl" = enum16{"HDF5 FLI Dataset", "Gate Image Folder", ".sdt FLI Dataset (Becker & Hickl)", ".ptu FLI Dataset (PicoQuant)", "SS1 FLI Dataset", "SS2 FLI Dataset", "I/m/phi Dataset", ".bin FLI Dataset (PicoQuant Binned)", ".bin FLI Dataset (Piccolo Binned)", ".mat FLI Dataset"}
  T37 = typedef "AlliGator Files.lvlib/AlliGator Data Series Type.ctl" = enum16{"Not a Supported Series", "Gate Images Folder Series", "SwissSPAD 2 Dataset Series", "B&H FLI Dataset Series", "PicoQuant PTU FLI Dataset Series", "PicoQuant BIN FLI Dataset Series", "Piccolo hist BIN FLI Dataset Series", "HDF5 FLI Dataset Series"}
  T38 = typedef "AlliGator Dual-Channel Datasets.lvlib/AlliGator Dataset Channel.ctl" = enum16{"G2", "INT"}
  T39 = typedef "AlliGator Settings.lvlib/AlliGator Gate Arithmetic.ctl" = enum16{"None", "INT-G2", "G2/INT*<INT>", "(1 - G2/INT)*<INT>"}
  T40 = typedef "AlliGator Source Image.lvlib/AlliGator Displayed Image.ctl" = enum16{"Single Gate", "Sum of All Gates", "Max of All Gates", "Min of All Gates", "-", "White Ligth Image", "Mask Image"}
  T41 = typedef "Image.lvlib/Named ROI Description.ctl" = cluster{"ROI Descriptor":T26, "ROI Name":string, "Overlay Color":u32}
  T42 = typedef "AlliGator Phasor Graph.lvlib/AlliGator Decay Metadata v3.ctl" = cluster{"ROI Descriptor":T26, "ROI Center":cluster{"X":i32, "Y":i32}, "Decay Background Subtraction Info":T43, "Decay Reverted":bool, "Decay Smoothened":bool, "Decay Straightened":bool, "Fitted Tau (Decay Straightening)":dbl, "Decay Shift Parameters":T45, "Decay Shifted":bool, "Decay Extrapolated":bool, "Decay Extrapolation Parameters":T47, "Decay Normalized":bool, "Fold Decay":bool, "# Folds":u32}
  T43 = typedef "AlliGator Decay Preprocessing.lvlib/AlliGator Decay Background Subtraction Info.ctl" = cluster{"Laser Period":dbl[unit], "Gate Duration":dbl[unit], "Baseline Subtraction Method":T44, "Background Definition Range":cluster{"Min Gate":dbl[unit], "Max Gate":dbl[unit]}, "Total Intensity w/o Bkgd Subtraction":dbl, "Bkgd-subtracted Intensity (exp)":dbl, "# Data Points":i32, "Background/Gate":dbl, "Fitted Lifetime":dbl[unit], "Bkgd-subtracted Intensity (theo)":dbl}
  T44 = typedef "AlliGator Decay Preprocessing.lvlib/AlliGator Baseline Subtraction Method.ctl" = enum16{"Mean", "Min", "Square Gated Single-Exponential", "File", "Constant"}
  T45 = typedef "XY Graph Add-Ons.lvlib/XY Graph Plot Shift Parameters.ctl" = cluster{"Type":T46, "Shift":dbl[unit], "Threshold":dbl, "Rotate":bool}
  T46 = typedef "XY Graph Add-Ons.lvlib/XY Graph Plot Shift Method.ctl" = enum16{"Default", "CFD", "Threshold", "Cross-Correlation"}
  T47 = typedef "AlliGator Decay Preprocessing.lvlib/AlliGator Decay Extrapolation Parameters.ctl" = cluster{"Additional Points":u32, "Head Fraction":dbl, "Fitted Tau":dbl, "Use Periodicity":bool, "Use Cursors":bool, "Tail Fraction":dbl}
  T48 = typedef "Phasor.lvlib/Calibration Phasor (m, phi).ctl" = cluster{"m":dbl, "phi":dbl, "Phasor Frequency":dbl[unit], "Reference Lifetime":dbl[unit]}
  T49 = typedef "Phasor.lvlib/Phasor Reference Series.ctl" = cluster{"m Array":dbl[], "phi Array":dbl[], "Phasor Frequency":dbl[unit], "Calibration Lifetime":dbl[unit]}
  T50 = typedef "Phasor.lvlib/Phasor Calibration Map v2.ctl" = cluster{"Phasor Frequency":dbl[unit], "Calibration Lifetime":dbl[unit], "ROI Centers":cluster{"X":i32, "Y":i32}[], "ROI Descriptors":T26[], "Map Resolution X":i32, "Map Resolution Y":i32, "z Array":cdb[]}
  T51 = typedef "Phasor.lvlib/Phasor (g, s).ctl" = cluster{"g":dbl, "s":dbl}
  T52 = typedef "AlliGator Phasor Graph.lvlib/AlliGator Raw Phasor Plot Data v5.ctl" = cluster{"Phasor Plot Name":string, "Raw Phasor Plot":T51[], "Phasor Frequency":dbl[unit], "[Decay Metadata]":T42[], "Raw Phasor Plot SDV":T51[], "Phasor SDV Options":T53, "[Calibration Phasor]":T48[], "Intensity Array":dbl[]}
  T53 = typedef "Phasor.lvlib/Phasor Standard Deviation Options.ctl" = cluster{"Compute Estimated SDV":bool, "# Replicas":u32, "Use Estimated Average Phasor":bool}
  T54 = typedef "AlliGator Phasor Plot.lvlib/AlliGator Phasor Multi-Harmonic Data.ctl" = cluster{"Base Frequency":dbl[unit], "# Harmonics":u8, "Harmonic Orders":u8[], "Phasor Plot Settings Checksum":u64, "Phasor Harmonic Data Array":T55[]}
  T55 = typedef "Phasor.lvlib/Phasor Harmonic Data.ctl" = cluster{"Phasor Harmonic Name":string, "Phasor Plot Settings Checksum":u64, "Phasor Frequency":dbl[unit], "Base Frequency":dbl[unit], "Harmonic Order":u8, "Phasor Plot Parameters":string, "Phasor Array [[CSG]]":csg[][], "Dataset File Path":path}
  T56 = typedef "AlliGator Decay Fit Parameter Map.lvlib/AlliGator Decay Fit Options & Parameters v4.ctl" = cluster{"SYNC Period":dbl[unit], "Fit Options":T57, "Fit Parameter Constraints":T64[], "MLE Baseline Offset":dbl, "MLE Baseline Offset Type":T66}
  T57 = typedef "Fits.lvlib/Decay Fit Options v4.ctl" = cluster{"Show Fit Residuals":bool, "Fit Model":T58, "Residual Type":T59, "Max Decay Percentile":dbl, "Min Decay Percentile":dbl, "Show Full Decay":bool, "Weights":T60, "Fitting Method":T61, "Compute Parameter Uncertainties":bool, "Periodic Boundaries":bool, "Model Calculation":T62, "Period":dbl[unit], "Termination Criteria":cluster{"Max Iterations":i32, "Max Function Calls":i32, "Max Time":dbl[unit], "Function Tolerance":dbl, "Parameter Tolerance":dbl, "Gradient Tolerance":dbl, "Min Lambda":dbl, "Max Lambda":dbl, "Initial Tick Count":u32}, "Offset Resolution":dbl[unit], "Use Local IRF":bool, "Fitting Algorithm":T63, "Show Confidence Interval ":bool, "Confidence Level":dbl}
  T58 = typedef "Fits.lvlib/Decay Model.ctl" = enum16{"1-Exponential", "2-Exponentials"}
  T59 = typedef "Fits.lvlib/Residual Type.ctl" = enum16{"Standard", "Normalized", "Reduced"}
  T60 = typedef "Fits.lvlib/Fit Weights Type v2.ctl" = enum16{"Unweighted", "1/Variance (Neyman)", "1/Variance (Pearson)", "Best of All"}
  T61 = typedef "Fits.lvlib/Non-linear Fitting Method v2.ctl" = enum16{"Least Square", "Least Absolute Residual", "Bisquare", "MLE", "-", "Best of All"}
  T62 = typedef "Fits.lvlib/Fit Calculation Method.ctl" = enum16{"Simulation", "Convolution", "Integration"}
  T63 = typedef "Fits.lvlib/Non-linear Fitting Algorithm.ctl" = enum16{"Levenberg-Marquardt", "Trust-Region Dogleg"}
  T64 = typedef "AlliGator Decay Fit.lvlib/AlliGator Decay Fit Parameter Constraints 2.ctl" = cluster{"Fit Parameter":T65, "Min Value":dbl, "Max Value":dbl, "Global":bool, "Used":bool}
  T65 = typedef "Fits.lvlib/Decay Fit Parameters In List.ctl" = enum16{"Offset", "Baseline", "A_1", "tau_1", "A_2", "tau_2"}
  T66 = typedef "Fits.lvlib/MLE Baseline Offset Type.ctl" = enum32{"Absolute", "Percentage"}
  T67 = typedef "AlliGator Decay Preprocessing.lvlib/AlliGator Decay Preprocessing Parameters.ctl" = cluster{"Background Subtraction":bool, "Straighten Decay":bool, "Reverse Gates":bool, "1-Normalized Decay":bool, "Smoothen Decay":bool, "Smoothing Parameter":dbl, "Shift Decay":bool, "Decay Shift Parameters":T45, "Extrapolate Decay":bool, "Additional Points":u32, "Head Fraction":dbl, "Pixel-Normalize Decay":bool, "Use Periodicity":bool, "Use Cursors":bool, "Tail Fraction":dbl, "Use Decay Pre-Processing":bool, "Fold Decay":bool, "# Folds":u32, "[0-1]-Normalized Decay":bool}
  T68 = typedef "Fits.lvlib/Decay Fit Parameters & Derived Quantities List v2.ctl" = enum16{"Offset", "Baseline", "A_1", "tau_1", "A_2", "tau_2", "<tau>_a", "f1_a", "f2_a", "<tau>_i", "f1_i", "f2_i", "-", "R^2", "Chi^2"}
  T69 = typedef "Fits.lvlib/Decay Fit Result Constraint.ctl" = cluster{"Fit Parameter":enum16{"Offset", "Baseline", "A_1", "tau_1", "A_2", "tau_2", "<tau>_a", "f1_a", "f2_a", "<tau>_i", "f1_i", "f2_i", "-", "R^2", "Chi^2", "Max Relative Residual", "<Residual ACF>", "Residual ACF SDV", "tau_2/tau_1"}, "Min Value":dbl, "Max Value":dbl, "Use Constraint":bool}
  T70 = typedef "AlliGator Decay Fit Parameter Map.lvlib/AlliGator Parameter Maps Data.ctl" = cluster{"Map Set Name":string, "[Parameter Names]":string[], "[[Parameters]]":dbl[][], "[[Parameter SDVs]]":dbl[][], "Decay Array Time Axis":dbl[], "[[IRFs]]":dbl[][], "IRF Array Time Axis":dbl[], "X Resolution":i32, "Y Resolution":i32, "Intensity Array":dbl[]}
  T71 = typedef "Image.lvlib/Image ROI Statistics Selection.ctl" = cluster{"Area (pixels)":bool, "% of Image":bool, "Total Intensity":bool, "Mean Intensity":bool, "Median Intensity":bool, "Mode Intensity":bool, "Intensity Standard Deviation":bool, "Min Intensity":bool, "Max Intensity":bool, "Mean SNR":bool, "Median SNR":bool, "Mode SNR":bool, "SNR Standard Deviation":bool, "Max SNR":bool, "Min SNR":bool, "# Rejected Pixels (NaN, Inf)":bool, "# Negative Pixels":bool, "Long Axis Length":bool, "Short Axis Length":bool, "Aspect Ratio":bool}
  T72 = cluster{"Global Rectangle":i32[], "Contours":cluster{"Contour Type":u32, "ROI Type":u32, "Points":i32[]}[]}
  T73 = typedef "Image.lvlib/Image Control ROI Description v2.ctl" = cluster{"Image Control Label":string, "Named ROI Description":T41}
  T74 = typedef "Image.lvlib/Image Display User Event Data.ctl" = cluster{"Image Control Refnum":T32, "Coords":T75, "button info":cluster{"button 1":bool, "button 2":bool, "button 3":bool, "button 4":bool}, "keys pressed":enum16{"0", "1", "2", "3", "4", "5", "6", "7", "8", "9", "A", "B", "C", "D", "E", "F", "G", "H", "I", "J", "K", "L", "M", "N", "O", "P", "Q", "R", "S", "T", "U", "V", "W", "X", "Y", "Z", "F1", "F2", "F3", "F4", "F5", "F6", "F7", "F8", "F9", "F10", "F11", "F12", "F13", "F14", "F15", "ADD", "BACK", "BACKSLASH", "CAPITAL", "COMMA", "DECIMAL", "DELETE", "DIVIDE", "DOWN", "END", "EQUALS", "ESCAPE", "GRAVE (`)", "HOME", "INSERT", "LBRACKET", "LCONTROL", "LEFT", "L ALT", "LSHIFT", "LWIN", "MINUS", "MULTIPLY", "NEXT", "NUMLOCK", "NUMPAD_0", "NUMPAD_1", "NUMPAD_2", "NUMPAD_3", "NUMPAD_4", "NUMPAD_5", "NUMPAD_6", "NUMPAD_7", "NUMPAD_8", "NUMPAD_9", "PAUSE", "PERIOD", "PRIOR (PG UP)", "RBRACKET", "RCONTROL", "RETURN", "RIGHT", "R ALT", "RSHIFT", "RWIN", "SCROLL", "SEMICOLON", "SLASH", "SPACE", "SUBTRACT", "TAB", "UP", "ENTER (num pad)", "' (quote)"}[]}
  T75 = typedef "LVPoint32TypeDef.ctl" = cluster{"Horizontal":i32, "Vertical":i32}
  T76 = typedef "AlliGator GUI.lvlib/AlliGator Image Mouse Up Event Data.ctl" = cluster{"Current ROI Tool":u32, "ROI Descriptor":T77, "Shift":bool, "Alt":bool, "Image Display Refnum":T32}
  T77 = typedef "Image.lvlib/Image ROI Descriptor.ctl" = cluster{"Global Rectangle":i32[], "Contours":T78[]}
  T78 = typedef "Image.lvlib/Image Contour Definition.ctl" = cluster{"Contour Type":T79, "ROI Type":T80, "Points":i32[]}
  T79 = typedef "Image.lvlib/Image Contour ID.ctl" = enum32{"External", "Internal"}
  T80 = typedef "Image.lvlib/Image ROI Type.ctl" = enum16{"No Selection", "Point", "Line", "Rectangle", "Oval", "Polygon", "Freehand Region", "Annulus", "Unused2", "Unused3", "Broken Line", "Freehand Line", "Rotated Rectangle"}
  T81 = typedef "Image.lvlib/Image Display Event.ctl" = cluster{"Item Tag":string, "Image Control Refnum":T32, "Coords":T75, "Item Path":string}
  T82 = typedef "AlliGator ROIs.lvlib/AlliGator ROI Selection Data.ctl" = cluster{"Action":T25, "ID":i32}
  T83 = typedef "Fits.lvlib/Decay Fit Parameters & Derived Quantities List.ctl" = enum16{"Offset", "Baseline", "A_1", "tau_1", "A_2", "tau_2", "<tau>_a", "f1_a", "f2_a", "<tau>_i", "f1_i", "f2_i", "-", "R^2", "Chi^2"}
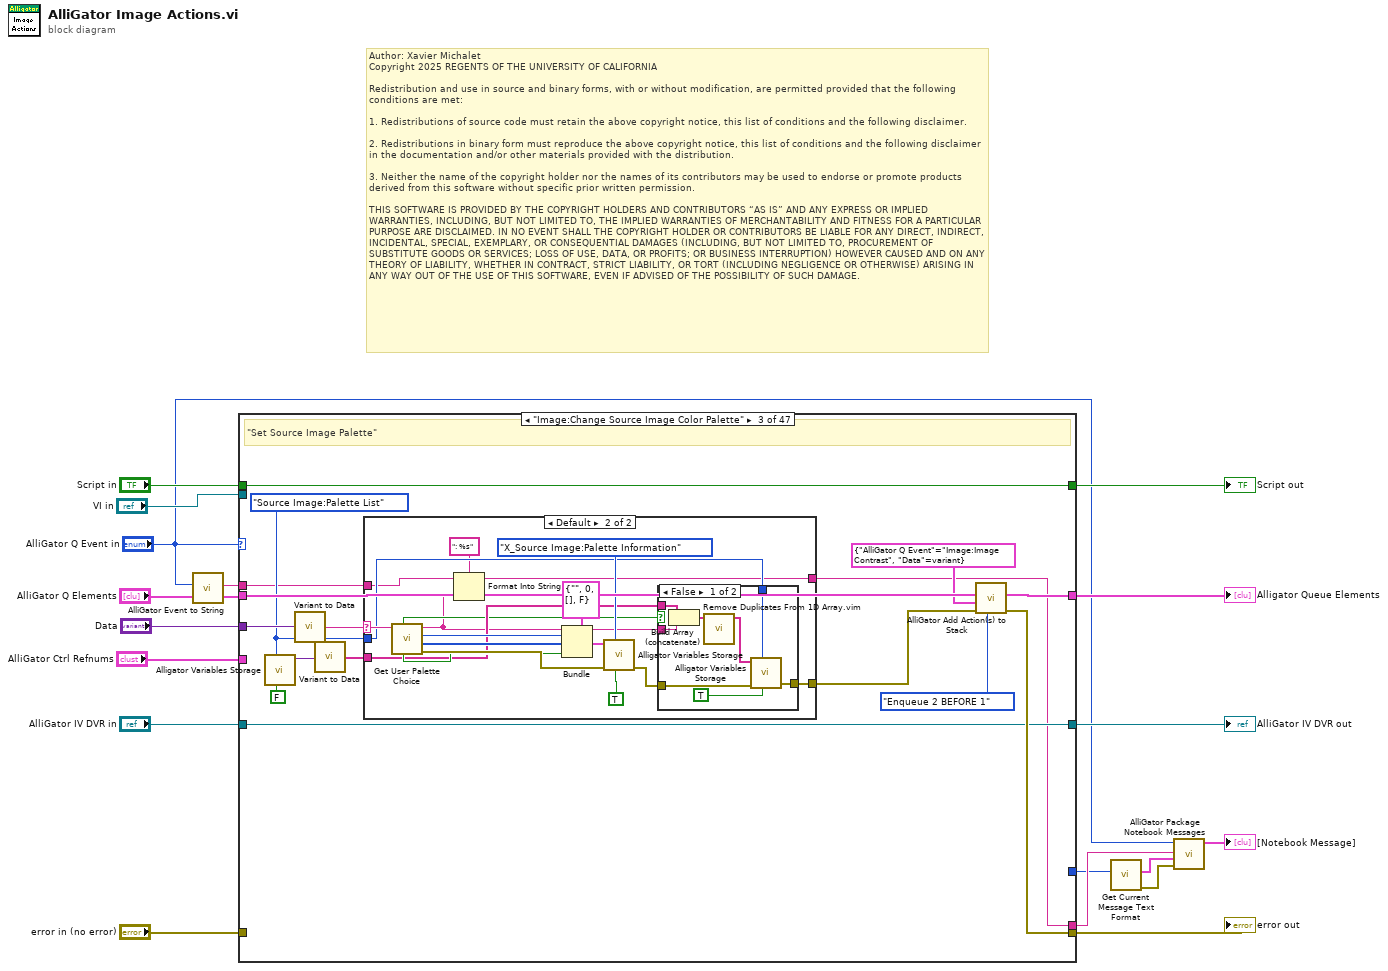
[diagram p0: block diagram]
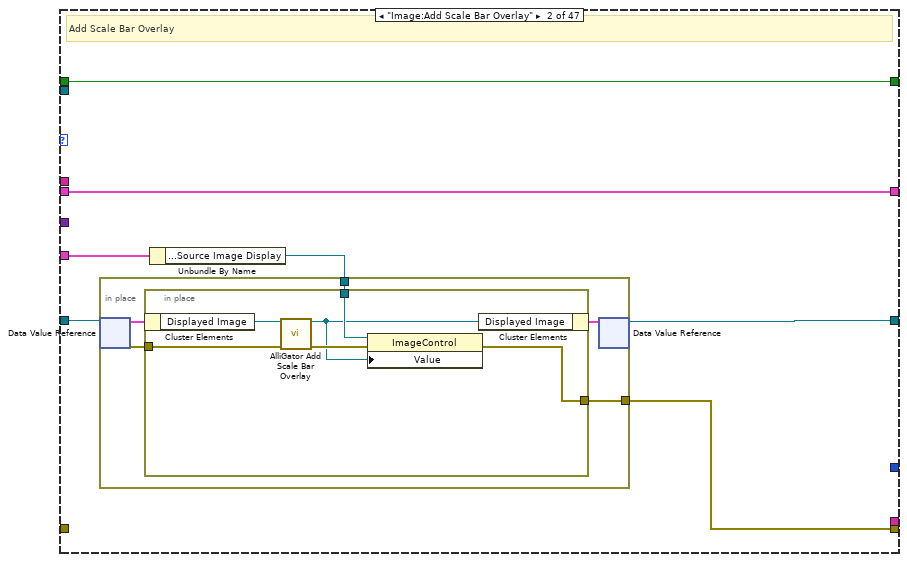
[diagram p3: hidden frame]
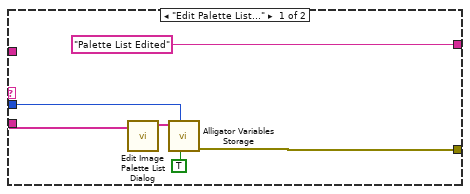
[diagram p4: hidden frame]
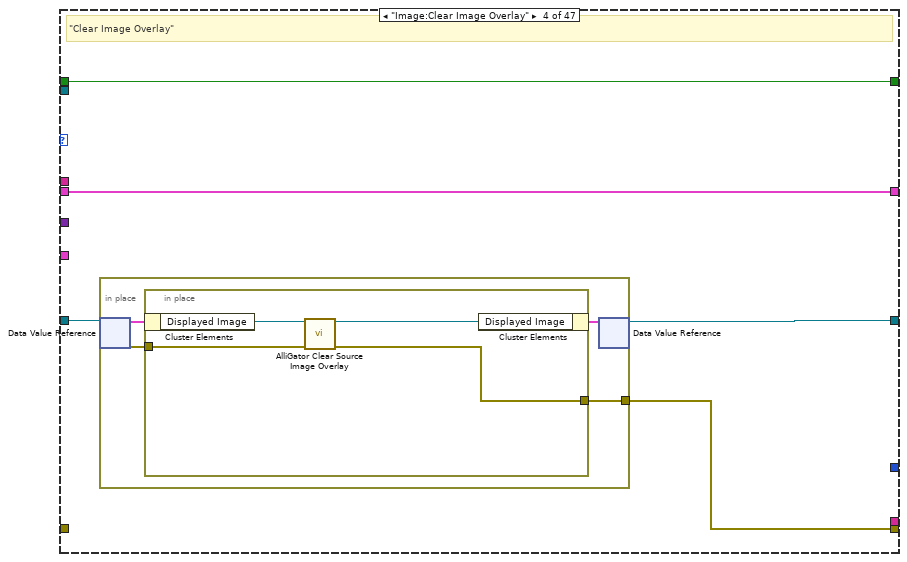
[diagram p6: hidden frame]
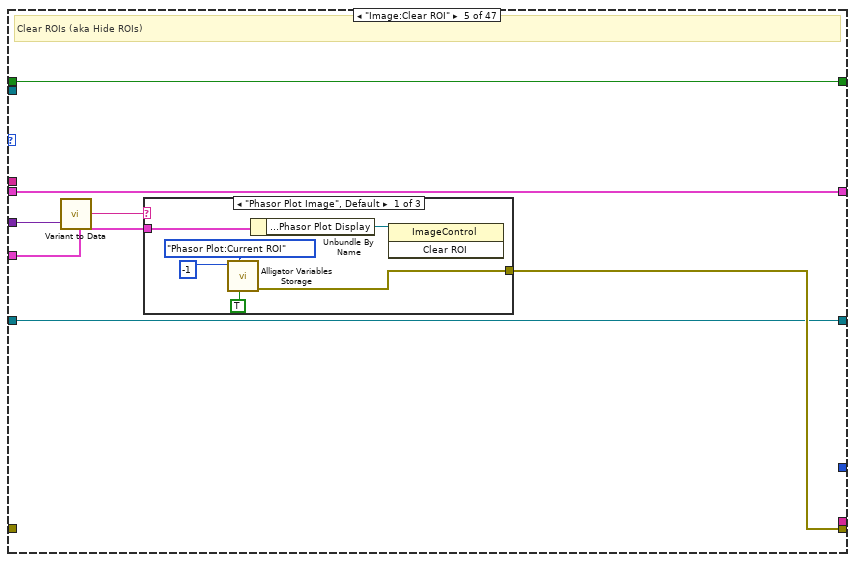
[diagram p7: hidden frame]
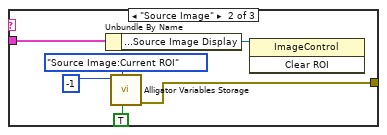
[diagram p8: hidden frame]
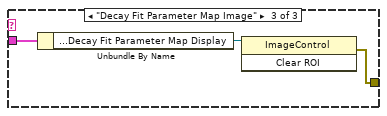
[diagram p9: hidden frame]
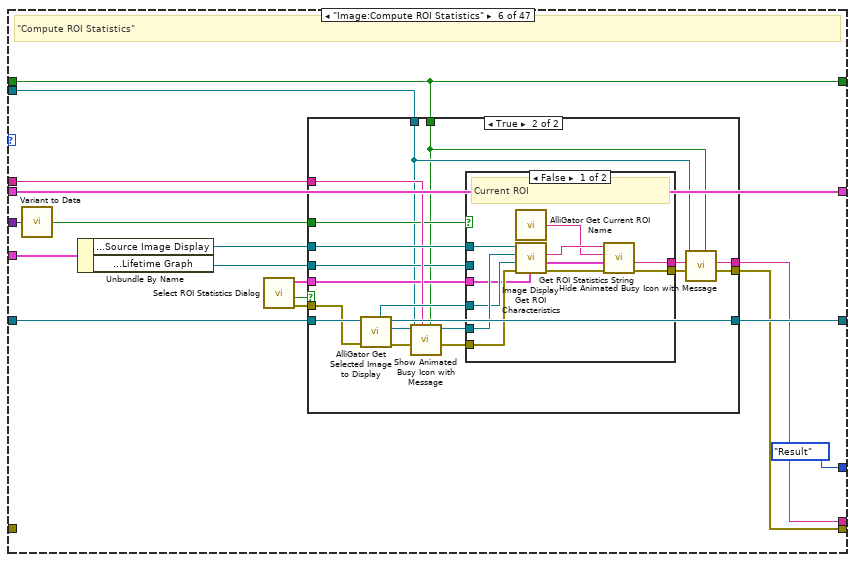
[diagram p10: hidden frame]
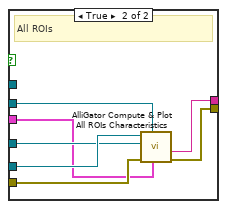
[diagram p12: hidden frame]
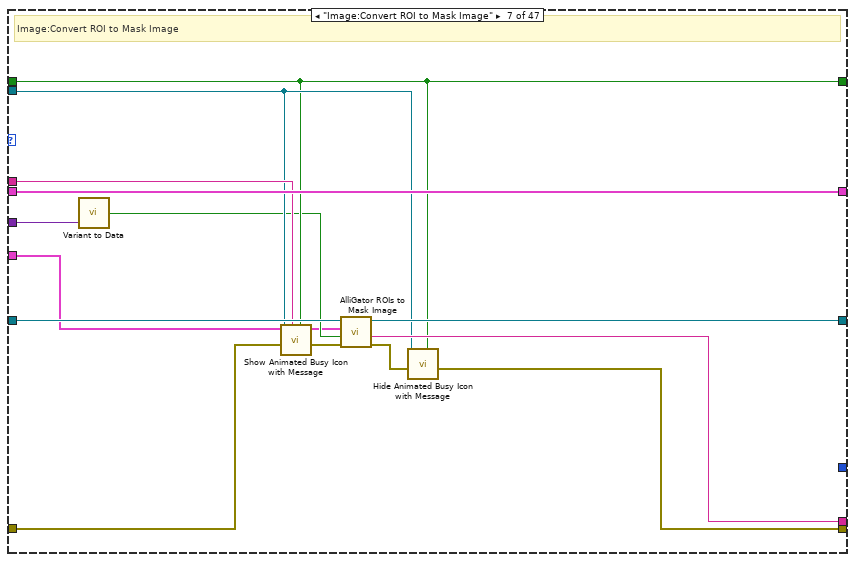
[diagram p13: hidden frame]
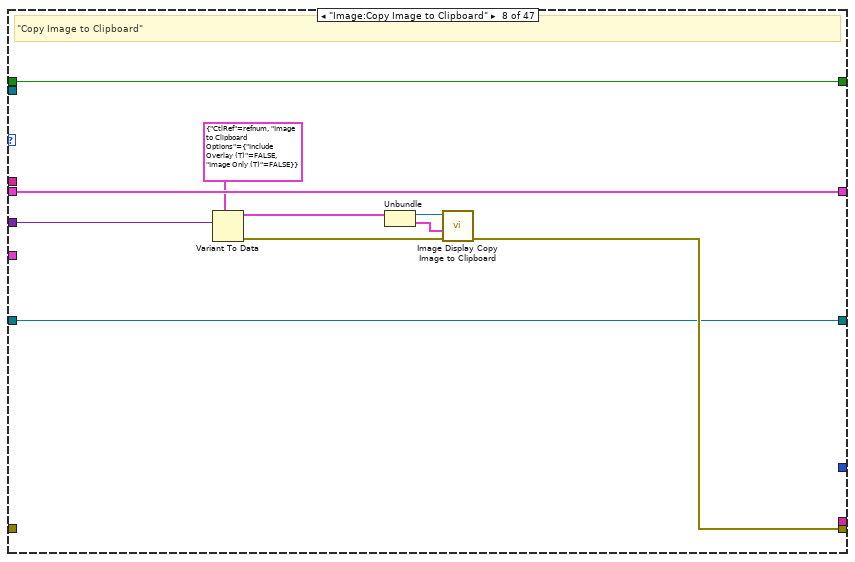
[diagram p14: hidden frame]
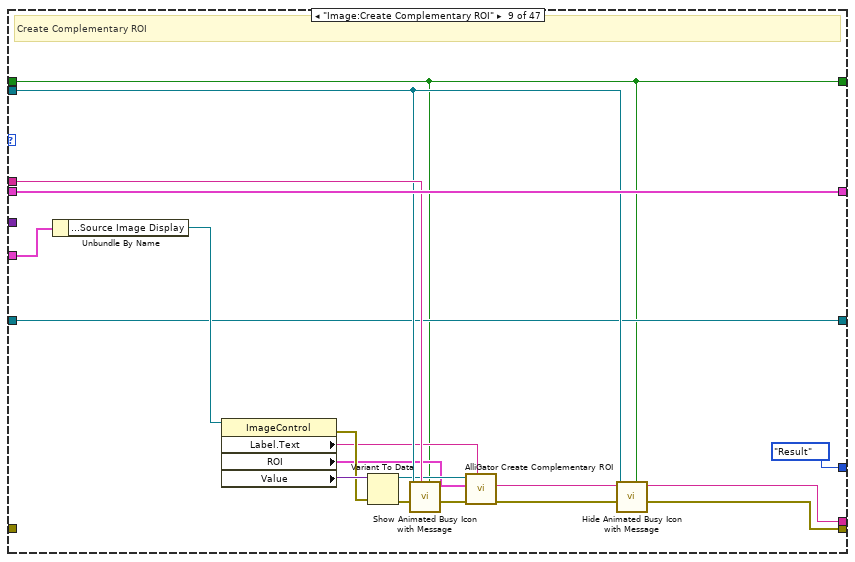
[diagram p15: hidden frame]
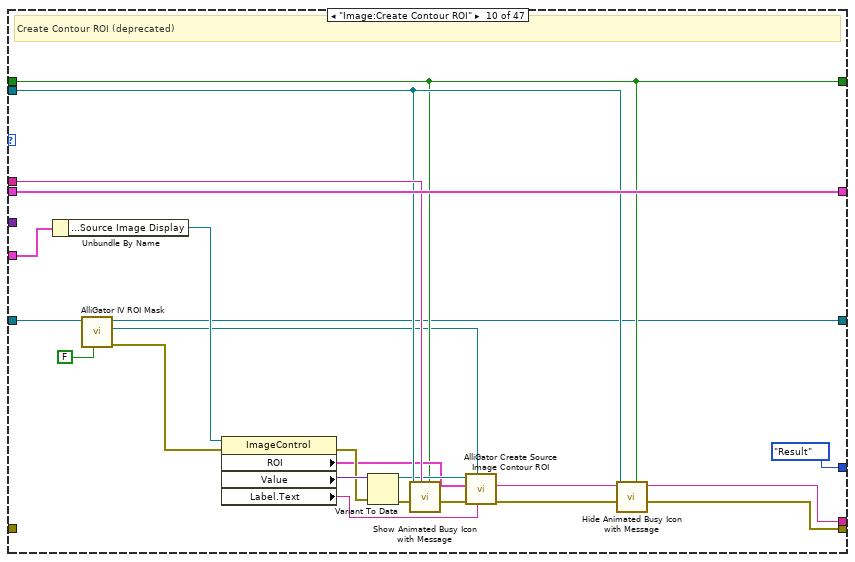
[diagram p16: hidden frame]
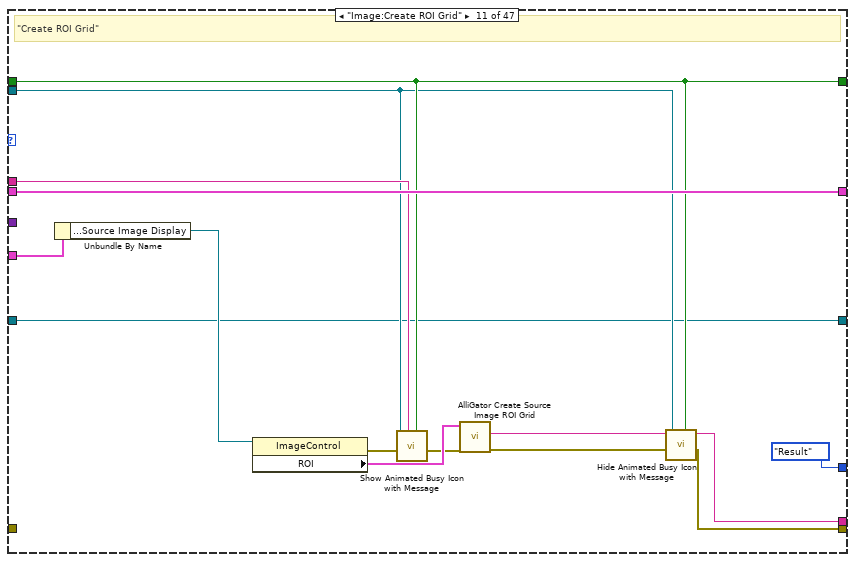
[diagram p17: hidden frame]
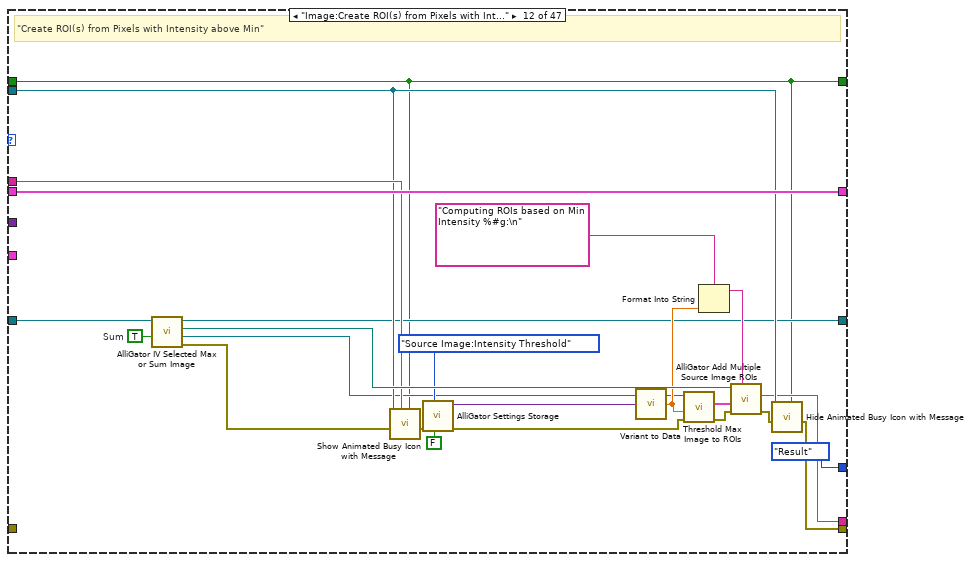
[diagram p18: hidden frame]
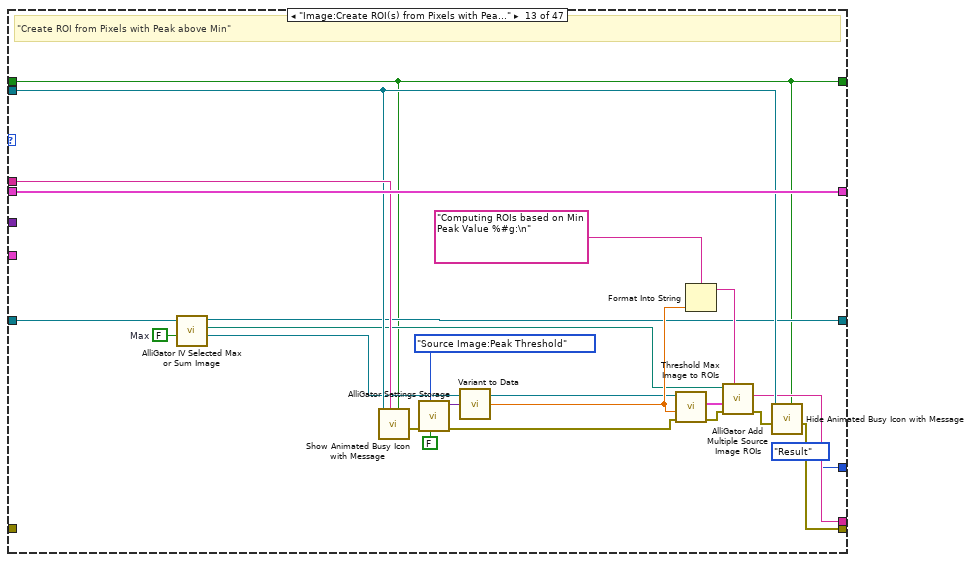
[diagram p19: hidden frame]
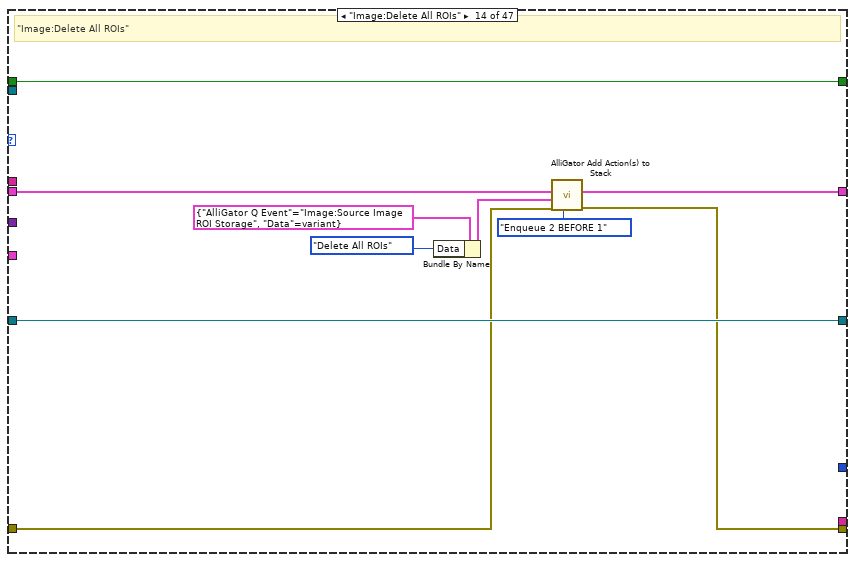
[diagram p20: hidden frame]
diagram:
  # "Author: Xavier Michalet\nCopyright 2025 REGENTS OF THE UNIVERSITY OF CALIFORNIA\n\nRedistribution and use in source and binary forms, with or without modification, are permitted provided that the following conditions are met:\n\n1. Redistributions of source code must retain the above copyright notice, this list of conditions and the following disclaimer.\n\n2. Redistributions in binary form must reproduce the above copyright notice, this list of conditions and the following disclaimer in the documentation and/or other materials provided with the distribution.\n\n3. Neither the name of the copyright holder nor the names of its contributors may be used to endorse or promote products derived from this software without specific prior written permission.\n\nTHIS SOFTWARE IS PROVIDED BY THE COPYRIGHT HOLDERS AND CONTRIBUTORS “AS IS” AND ANY EXPRESS OR IMPLIED WARRANTIES, INCLUDING, BUT NOT LIMITED TO, THE IMPLIED WARRANTIES OF MERCHANTABILITY AND FITNESS FOR A PARTICULAR PURPOSE ARE DISCLAIMED. IN NO EVENT SHALL THE COPYRIGHT HOLDER OR CONTRIBUTORS BE LIABLE FOR ANY DIRECT, INDIRECT, INCIDENTAL, SPECIAL, EXEMPLARY, OR CONSEQUENTIAL DAMAGES (INCLUDING, BUT NOT LIMITED TO, PROCUREMENT OF SUBSTITUTE GOODS OR SERVICES; LOSS OF USE, DATA, OR PROFITS; OR BUSINESS INTERRUPTION) HOWEVER CAUSED AND ON ANY THEORY OF LIABILITY, WHETHER IN CONTRACT, STRICT LIABILITY, OR TORT (INCLUDING NEGLIGENCE OR OTHERWISE) ARISING IN ANY WAY OUT OF THE USE OF THIS SOFTWARE, EVEN IF ADVISED OF THE POSSIBILITY OF SUCH DAMAGE."
  n1 = call "AlliGator Event to String.vi"("AlliGator Q Event"="AlliGator Q Event in") -> ("String"=w8:string)  [unwired: 8 in]
  n2 = case shown="\"Image:Change Source Image Color Palette\"" "AlliGator Q Event in" {
    tunnel: "Data" -> [_ _ w56 _ w108 w131 w187 w200 _ _ _ _ _ _ _ _ _ _ w387 w407 w416 _ w470 w534 _ w550 w564 _ _ w613 w630 w681 w702 w746 w786 w828 w832 _ w854 _ w885 w901 _ _ _ w941 _]
    tunnel: "AlliGator Q Elements" -> [w22 w29 w55 w94 w109 w141 w191 w201 w219 w241 w255 w279 w302 w312 w322 w330 w346 w360 w388 w411 w446 w466 w480 w535 w545 w552 w562 w573 w587 w608 w640 w685 w723 w749 w801 w829 w836 w849 w858 w870 w879 w905 w915 w930 w937 w944 w951]
    tunnel: [w22 w29 w54 w94 w109 w141 w191 w201 w219 w241 w255 w279 w302 w309 w319 w330 w343 w360 w388 w411 w446 w464 w480 w535 w542 w551 w561 w573 w587 w607 w640 w685 w723 w749 w801 w829 w836 w849 w858 w870 w877 w905 w912 w930 w937 w944 w951] -> w10
    tunnel: "VI in" -> [_ _ _ _ _ w133 w181 _ w213 w235 w245 w264 w288 _ _ _ _ w348 w369 w400 w428 _ w479 w526 _ _ _ _ _ w609 w628 w661 w704 w739 w772 w815 _ _ _ w868 w881 _ _ w917 _ _ _]
    tunnel: [w21 w28 w49 w93 w106 w132 w180 w194 w203 w226 w249 w257 w281 w311 w321 w329 w345 w347 w368 w399 w421 w469 w478 w523 w544 w554 w566 w572 w586 w597 w619 w660 w703 w731 w771 w814 w835 w844 w857 w867 w880 w904 w914 w916 w936 w943 w950] -> w11
    tunnel: "Script in" -> [w21 w28 w49 w93 w106 w132 w180 w194 w203 w226 w249 w257 w281 w311 w321 w329 w345 w347 w368 w399 w421 w469 w478 w523 w544 w554 w566 w572 w586 w597 w619 w660 w703 w731 w771 w814 w835 w844 w857 w867 w880 w904 w914 w916 w936 w943 w950]
    tunnel: w8 -> [_ _ w41 _ _ w135 w183 _ w217 w239 w247 w275 w298 _ _ _ _ w352 w371 w402 w427 _ w473 w521 _ _ _ _ _ w610 w634 w663 w705 w738 w773 w817 _ _ _ w866 _ _ _ w918 _ _ _]
    tunnel: "error in (no error)" -> [w20 _ _ _ _ _ w185 _ _ _ _ _ _ w304 w314 w324 w338 w354 _ w404 _ w468 _ w522 w537 w546 w563 w567 _ _ _ _ _ _ _ w810 w834 _ w856 w869 _ _ w907 w921 _ w938 w945]
    tunnel: [w20 w25 w48 w90 w105 w134 w182 w193 w215 w237 w250 w276 w299 w303 w313 w325 w337 w349 w370 w401 w445 w468 w477 w528 w536 w547 w560 w568 w579 w604 w632 w665 w713 w747 w781 w816 w834 w840 w856 w869 w871 w895 w906 w919 w935 w939 w948] -> w1
    tunnel: "AlliGator Ctrl Refnums" -> [_ w24 _ _ w104 w139 w178 _ w216 w238 w246 _ _ _ _ _ _ _ w376 _ w429 _ w475 _ _ _ w557 w569 w578 _ w633 w671 w715 _ w783 w813 _ w839 w851 w861 w875 w897 _ w928 w933 _ w949]
    tunnel: "AlliGator IV DVR in" -> [w19 w27 w47 w92 w103 w138 w189 w192 w211 w233 w244 w261 w287 w310 w320 w328 w344 w358 w379 w409 w426 w467 w472 w525 w543 w553 w565 w571 w575 w602 w625 w668 w689 w730 w770 w820 w833 w838 w855 w865 w883 w887 w913 w925 w932 w942 w947]
    tunnel: [w19 w26 w47 w91 w103 w137 w188 w192 w211 w224 w244 w262 w285 w310 w320 w328 w344 w357 w379 w408 w425 w467 w471 w525 w543 w553 w565 w570 w575 w601 w623 w667 w688 w729 w767 w820 w833 w838 w855 w864 w883 w887 w913 w924 w932 w942 w946] -> w18
    tunnel: [_ _ w46 _ _ w136 w186 _ w210 w232 w243 w258 w282 _ _ w323 _ w353 w378 w405 _ _ _ w524 _ _ _ _ w574 w598 w621 w666 w708 w732 w776 w819 _ w837 _ _ _ w886 _ _ w931 _ _] -> w5
    tunnel: [_ _ _ _ _ Text_Format_List."Result" ("Text Format") _ _ Text_Format_List."Result" ("Text Format") Text_Format_List."Result" ("Text Format") Text_Format_List."Result" ("Text Format") Text_Format_List."Result" ("Text Format") Text_Format_List."Result" ("Text Format") _ _ _ _ _ Text_Format_List."Result" ("Text Format") _ _ _ _ _ _ _ Text_Format_List."Message" ("Text Format") _ _ Text_Format_List."Result" ("Text Format") Text_Format_List."Result" ("Text Format") _ _ _ _ _ _ _ _ _ _ _ _ _ _ _ _] -> w3
    frame "---- Image ----", Default {
    }
    frame "Image:Add Scale Bar Overlay" {
      # "Add Scale Bar Overlay"
      n3 = Unbundle By Name(w24) -> ("Registered Events Ctrl Refnums.Source Image Display"=w23:refnum<vi>)
      n4 = in-place "In Place Element Structure" {
        in-place-border: [w31] -> w25
        in-place-border: w23 -> [w30]
        n5 = in-place-dvr #1 ("Data Value Reference Read / Write Element")(w27) -> (w34:T34, w32:errorcluster)
        n6 = in-place "In Place Element Structure" {
          in-place-border: w32 -> [w39]
          in-place-border: [w36] -> w31
          in-place-border: w30 -> [w38]
          n7 = in-place-cluster #2 ("Unbundle / Bundle Elements")(w34) -> ("Displayed Image"=w40:T28)
          n8 = call "AlliGator Add Scale Bar Overlay.vi"("Source Image in"=w40, "Error In"=w39) -> ("Source Image out"=w35:T28, "Error Out"=w37:errorcluster)  [unwired: 12 in]
          n9 = property class="ImageControl"(reference=w38, error in=w37, "Value"=w35) -> (error out=w36:errorcluster)  [unwired: 1 out]
          n10 = in-place-cluster #2 ("Unbundle / Bundle Elements")("Displayed Image"=w35) -> (w33:T34)
        }
        n11 = in-place-dvr #1 ("Data Value Reference Read / Write Element")(w33) -> (w26:refnum<data-value>)  [unwired: 1 out]
      }
    }
    frame "Image:Change Source Image Color Palette" {
      w44 = AlliGator_Variables_List."Source Image:Palette List" ("Alligator Variable")
      # "\"Set Source Image Palette\""
      n12 = call "Alligator Variables Storage.vi"("Get(F)/Set"=FALSE, "AlliGator Variable"=w44) -> ("Data out"=w43:variant)  [unwired: 7 in, 2 out]
      n13 = call-poly "Variant to Data.vi"("Variant"=w56) -> ("String"=w53:string)  [unwired: 8 in]
      n14 = call-poly "Variant to Data.vi"("Variant"=w43) -> ("String Array"=w42:string[])  [unwired: 8 in]
      n15 = case shown="Default" w53 {
        selector: w53 -> [_ w80]
        tunnel: [w60 w70] -> w51
        tunnel: ["Palette List Edited" ("Append to Message") w66] -> w46
        tunnel: w44 -> [w58 w68]
        tunnel: w42 -> [w57 w69]
        tunnel: w41 -> [_ w64]
        frame "Edit Palette List..." {
          n16 = call "Edit Image Palette List Dialog.vi"("Palette List (in)"=w57) -> ("Palette List (out)"=w62:string[])  [unwired: 10 in]
          n17 = call "Alligator Variables Storage.vi"("Get(F)/Set"=TRUE, "AlliGator Variable"=w58, "Data in"=w62) -> ("Error Out"=w60:errorcluster)  [unwired: 6 in, 2 out]
        }
        frame Default {
          n18 = call "Get User Palette Choice.vi"("Palette"=w80) -> ("Error Out"=w74:errorcluster, "Palette Colors"=w78:u32[], "Palette Type"=w79:T20, "Palette Name (# Colors)"=w65:string, "Interpolate?"=w73:bool, "Built-in Palette?"=w67:bool)  [unwired: 3 in, 2 out]
          n19 = Format Into String(format string=": %s", initial string=w64, w65) -> (resulting string=w66:string)  [unwired: 1 in, 1 out]
          n20 = Bundle(cluster=T19 {"Palette Name [# Colors,int?,inv?]"="", "Palette Type"=0, "Palette Colors"=[], "Interpolate?"=FALSE} ("Image Display Palette Information"), "Palette Name [# Colors,int?,inv?]"=w65, "Palette Type"=w79, "Palette Colors"=w78, "Interpolate?"=w73) -> (w76:T19)
          n21 = call "Alligator Variables Storage.vi"("Get(F)/Set"=TRUE, "AlliGator Variable"=AlliGator_Variables_List."X_Source Image:Palette Information" ("Alligator Variable"), "Error In"=w74, "Data in"=w76) -> ("Error Out"=w71:errorcluster)  [unwired: 5 in, 2 out]
          n22 = case shown="False" w67 {
            tunnel: w71 -> [w88 w89]
            tunnel: [w87 w89] -> w70
            tunnel: w65 -> [w86 _]
            tunnel: w69 -> [w85 _]
            tunnel: w68 -> [w83 _]
            frame False {
              n23 = Build Array (concatenate)(w85, w86) -> (w84:string[])
              n24 = call "Remove Duplicates From 1D Array.vim"("array"=w84) -> ("array with duplicates removed"=w82:string[])  [unwired: 10 in]
              n25 = call "Alligator Variables Storage.vi"("Get(F)/Set"=TRUE, "AlliGator Variable"=w83, "Error In"=w88, "Data in"=w82) -> ("Error Out"=w87:errorcluster)  [unwired: 5 in, 2 out]
            }
            frame True {
            }
          }
        }
      }
      n26 = call-poly "AlliGator Add Action(s) to Stack.vi"("Elements Order in Action Stack (Default: 2 BEFORE 1)"=Alligator_Elements_Order_in_Action_Stack."Enqueue 2 BEFORE 1", "Error In"=w51, "Alligator Atomic Action"=T6 {"AlliGator Q Event"=enum."Image:Image Contrast", "Data"=variant}, "Alligator Queue Element 1"=w55) -> ("Error Out"=w48:errorcluster, "Alligator Queue Element 1 (+ 2)"=w54:T6[])  [unwired: 6 in]
    }
    frame "Image:Clear Image Overlay" {
      # "\"Clear Image Overlay\""
      n27 = in-place "In Place Element Structure" {
        in-place-border: [w95] -> w90
        n28 = in-place-dvr #3 ("Data Value Reference Read / Write Element")(w92) -> (w98:T34, w96:errorcluster)
        n29 = in-place "In Place Element Structure" {
          in-place-border: w96 -> [w100]
          in-place-border: [w99] -> w95
          n30 = in-place-cluster #4 ("Unbundle / Bundle Elements")(w98) -> ("Displayed Image"=w102:T28)
          n31 = call "AlliGator Clear Source Image Overlay.vi"("Source Image in"=w102, "Error In"=w100) -> ("Source Image out"=w101:T28, "Error Out"=w99:errorcluster)  [unwired: 12 in]
          n32 = in-place-cluster #4 ("Unbundle / Bundle Elements")("Displayed Image"=w101) -> (w97:T34)
        }
        n33 = in-place-dvr #3 ("Data Value Reference Read / Write Element")(w97) -> (w91:refnum<data-value>)  [unwired: 1 out]
      }
    }
    frame "Image:Clear ROI" {
      # "Clear ROIs (aka Hide ROIs)"
      n34 = call-poly "Variant to Data.vi"("Variant"=w108) -> ("String"=w107:string)  [unwired: 8 in]
      n35 = case shown="\"Phasor Plot Image\", Default" w107 {
        tunnel: [w112 w118 w122] -> w105
        tunnel: w104 -> [w111 w116 w123]
        frame "Phasor Plot Image", Default {
          n36 = call "Alligator Variables Storage.vi"("Get(F)/Set"=TRUE, "AlliGator Variable"=AlliGator_Variables_List."Phasor Plot:Current ROI" ("Alligator Variable"), "Data in"=-1 ("Current ROI")) -> ("Error Out"=w112:errorcluster)  [unwired: 6 in, 2 out]
          n37 = Unbundle By Name(w111) -> ("Registered Events Ctrl Refnums.Phasor Plot Display"=w110:refnum<vi>)
          n38 = invoke on="Invoke Node" class="ImageControl" method="Clear ROI"(reference=w110) -> ()  [unwired: 2 in, 3 out]
        }
        frame "Source Image" {
          n39 = Unbundle By Name(w116) -> ("Registered Events Ctrl Refnums.Source Image Display"=w117:refnum<vi>)
          n40 = call "Alligator Variables Storage.vi"("Get(F)/Set"=TRUE, "AlliGator Variable"=AlliGator_Variables_List."Source Image:Current ROI" ("Alligator Variable"), "Data in"=-1 ("Current ROI")) -> ("Error Out"=w118:errorcluster)  [unwired: 6 in, 2 out]
          n41 = invoke on="Invoke Node" class="ImageControl" method="Clear ROI"(reference=w117) -> ()  [unwired: 2 in, 3 out]
        }
        frame "Decay Fit Parameter Map Image" {
          n42 = Unbundle By Name(w123) -> ("Registered Events Ctrl Refnums.Decay Fit Parameter Map Display"=w124:refnum<vi>)
          n43 = invoke on="Invoke Node" class="ImageControl" method="Clear ROI"(reference=w124) -> (error out=w122:errorcluster)  [unwired: 2 in, 2 out]
        }
      }
    }
    frame "Image:Compute ROI Statistics" {
      # "\"Compute ROI Statistics\""
      n44 = call-poly "Variant to Data.vi"("Variant"=w131) -> ("Value"=w130:bool)  [unwired: 8 in]
      n45 = Unbundle By Name(w139) -> ("Registered Events Ctrl Refnums.Source Image Display"=w140:refnum<vi>, "Registered Events Ctrl Refnums.Lifetime Graph"=w129:refnum<vi>)
      n46 = call "Select ROI Statistics Dialog.vi"() -> ("error out"=w126:errorcluster, "OK?"=w128:bool, "ROI Statistics out"=w127:T71)  [unwired: 9 in]
      n47 = case shown="True" w128 {
        tunnel: w140 -> [_ w158]
        tunnel: w138 -> [w142 w156]
        tunnel: [w142 w155] -> w137
        tunnel: [_ w152] -> w136
        tunnel: w135 -> [_ w150]
        tunnel: [_ w149] -> w134
        tunnel: w133 -> [_ w144]
        tunnel: w132 -> [_ w143]
        tunnel: w130 -> [_ w148]
        tunnel: w129 -> [_ w147]
        tunnel: w127 -> [_ w145]
        tunnel: w126 -> [_ w146]
        frame False {
        }
        frame True {
          n48 = call "AlliGator Get Selected Image to Display.vi"("Error In"=w146, "AlliGator IV DVR in"=w156) -> ("Error Out"=w154:errorcluster, "Image out"=w157:T28, "AlliGator IV DVR out"=w155:refnum<data-value>, "ROI Mask"=w153:T28)  [unwired: 4 in, 2 out]
          n49 = call "Show Animated Busy Icon with Message.vi"("Already active? (F)"=w143, "Message"=w150, "Error In"=w154, "Target VI Refnum"=w144) -> ("Error Out"=w151:errorcluster)  [unwired: 7 in]
          n50 = case shown="False" w148 {
            tunnel: [w169 w176] -> w159
            tunnel: w158 -> [w167 _]
            tunnel: w157 -> [w166 w175]
            tunnel: w153 -> [w164 w174]
            tunnel: [w163 w172] -> w152
            tunnel: w151 -> [w162 w177]
            tunnel: w147 -> [_ w173]
            tunnel: w145 -> [w160 w171]
            frame False {
              # "Current ROI"
              n51 = call "AlliGator Get Current ROI Name.vi"() -> ("Current ROI Name"=w161:string)  [unwired: 9 in]
              n52 = call "Image Display Get ROI Characteristics.vi"("ROI Characteristics Selection"=w160, "Error In"=w162, "ROI Mask refnum"=w164, "Image refnum"=w166, "Image Control Refnum"=w167) -> ("Error Out"=w170:errorcluster, "ROI"=w168:T72, "ROI Characteristics String"=w165:string)  [unwired: 3 in, 1 out]
              n53 = call "Get ROI Statistics String.vi"("error in (no error)"=w170, "ROI"=w168, "ROI Name (\"\")"=w161, "ROI Statistics String"=w165) -> ("error out"=w169:errorcluster, "Message"=w163:string)  [unwired: 6 in]
            }
            frame True {
              # "All ROIs"
              n54 = call "AlliGator Compute & Plot All ROIs Characteristics.vi"("ROI Statistics Selection"=w171, "Lifetime Graph"=w173, "error in (no error)"=w177, "ROI Mask Refnum"=w174, "Source Image Refnum"=w175) -> ("error out"=w176:errorcluster, "ROI Statistics String"=w172:string)  [unwired: 5 in]
            }
          }
          n55 = call "Hide Animated Busy Icon with Message.vi"("Already active? (F)"=w143, "Error In"=w159, "Target VI reference"=w144) -> ("Error Out"=w149:errorcluster)  [unwired: 8 in]
        }
      }
    }
    frame "Image:Convert ROI to Mask Image" {
      # "Image:Convert ROI to Mask Image"
      n56 = call-poly "Variant to Data.vi"("Variant"=w187) -> ("Value"=w179:bool)  [unwired: 8 in]
      n57 = call "Show Animated Busy Icon with Message.vi"("Already active? (F)"=w180, "Message"=w183, "Error In"=w185, "Target VI Refnum"=w181) -> ("Error Out"=w184:errorcluster)  [unwired: 7 in]
      n58 = call "AlliGator ROIs to Mask Image.vi"("error in"=w184, "All ROIs?"=w179, "AlliGator Ctrl Refnums"=w178, "Data Value Reference in"=w189) -> ("error out"=w190:errorcluster, "Message"=w186:string, "Data Value Reference out"=w188:refnum<data-value>)  [unwired: 5 in]
      n59 = call "Hide Animated Busy Icon with Message.vi"("Already active? (F)"=w180, "Error In"=w190, "Target VI reference"=w181) -> ("Error Out"=w182:errorcluster)  [unwired: 8 in]
    }
    frame "Image:Copy Image to Clipboard" {
      # "\"Copy Image to Clipboard\""
      n60 = Variant To Data(type=T23 {"CtlRef"=refnum, "Image to Clipboard Options"={"Include Overlay (T)"=FALSE, "Image Only (T)"=FALSE}} ("output cluster"), Variant=w200) -> (data=w199:T23, error out=w198:errorcluster)  [unwired: 1 in]
      n61 = Unbundle(w199) -> ("CtlRef"=w196:refnum<vi>, "Image to Clipboard Options"=w195:T22)
      n62 = call "Image Display Copy Image to Clipboard.vi"("Error In"=w198, "Image to Clipboard Options"=w195, "Display Image Control Refnum"=w196) -> ("Error Out"=w193:errorcluster)  [unwired: 8 in]
    }
    frame "Image:Create Complementary ROI" {
      # "Create Complementary ROI"
      n63 = Unbundle By Name(w216) -> ("Registered Events Ctrl Refnums.Source Image Display"=w218:refnum<vi>)
      n64 = property on="Property Node" class="ImageControl"(reference=w218) -> (error out=w208:errorcluster, "Label.Text"=w204:string, "ROI"=w205:T72, "Value"=w209:variant)  [unwired: 1 in, 1 out]
      n65 = Variant To Data(error in=w208, Variant=w209) -> (data=w206:T28, error out=w207:errorcluster)  [unwired: 1 in]
      n66 = call "Show Animated Busy Icon with Message.vi"("Already active? (F)"=w203, "Message"=w217, "Error In"=w207, "Target VI Refnum"=w213) -> ("Error Out"=w212:errorcluster)  [unwired: 7 in]
      n67 = call "AlliGator Create Complementary ROI.vi"("Image Label"=w204, "Error In"=w212, "ROI"=w205, "Image"=w206) -> ("Error Out"=w214:errorcluster, "Message"=w210:string)  [unwired: 6 in]
      n68 = call "Hide Animated Busy Icon with Message.vi"("Already active? (F)"=w203, "Error In"=w214, "Target VI reference"=w213) -> ("Error Out"=w215:errorcluster)  [unwired: 8 in]
    }
    frame "Image:Create Contour ROI" {
      # "Create Contour ROI (deprecated)"
      n69 = Unbundle By Name(w238) -> ("Registered Events Ctrl Refnums.Source Image Display"=w240:refnum<vi>)
      n70 = call "AlliGator IV ROI Mask.vi"("Get (F)/ Set (T)"=FALSE, "AlliGator IV DVR in"=w233) -> ("error out"=w221:errorcluster, "ROI Mask Image"=w222:T28, "AlliGator IV DVR out"=w224:refnum<data-value>)  [unwired: 7 in]
      n71 = property on="Property Node" class="ImageControl"(reference=w240, error in=w221) -> (error out=w230:errorcluster, "ROI"=w227:T72, "Value"=w231:variant, "Label.Text"=w225:string)  [unwired: 1 out]
      n72 = Variant To Data(error in=w230, Variant=w231) -> (data=w228:T28, error out=w229:errorcluster)  [unwired: 1 in]
      n73 = call "Show Animated Busy Icon with Message.vi"("Already active? (F)"=w226, "Message"=w239, "Error In"=w229, "Target VI Refnum"=w235) -> ("Error Out"=w234:errorcluster)  [unwired: 7 in]
      n74 = call "AlliGator Create Source Image Contour ROI.vi"("Image Label"=w225, "ROI Mask"=w222, "Error In"=w234, "ROI"=w227, "Image"=w228) -> ("Error Out"=w236:errorcluster, "Message"=w232:string)  [unwired: 5 in]
      n75 = call "Hide Animated Busy Icon with Message.vi"("Already active? (F)"=w226, "Error In"=w236, "Target VI reference"=w235) -> ("Error Out"=w237:errorcluster)  [unwired: 8 in]
    }
    frame "Image:Create ROI Grid" {
      # "\"Create ROI Grid\""
      n76 = Unbundle By Name(w246) -> ("Registered Events Ctrl Refnums.Source Image Display"=w248:refnum<vi>)
      n77 = property on="Property Node" class="ImageControl"(reference=w248) -> (error out=w253:errorcluster, "ROI"=w254:T72)  [unwired: 1 in, 1 out]
      n78 = call "Show Animated Busy Icon with Message.vi"("Already active? (F)"=w249, "Message"=w247, "Error In"=w253, "Target VI Refnum"=w245) -> ("Error Out"=w251:errorcluster)  [unwired: 7 in]
      n79 = call "AlliGator Create Source Image ROI Grid.vi"("Error In"=w251, "ROI"=w254) -> ("Error Out"=w252:errorcluster, "Message"=w243:string)  [unwired: 8 in]
      n80 = call "Hide Animated Busy Icon with Message.vi"("Already active? (F)"=w249, "Error In"=w252, "Target VI reference"=w245) -> ("Error Out"=w250:errorcluster)  [unwired: 8 in]
    }
    frame "Image:Create ROI(s) from Pixels with Intensity above Min_Scriptable" {
      w259 = TRUE  # Sum
      # "\"Create ROI(s) from Pixels with Intensity above Min\""
      n81 = call "AlliGator IV Selected Max or Sum Image.vi"("Sum (T)/ Max (F)"=w259, "AlliGator IV DVR in"=w261) -> ("Error Out"=w260:errorcluster, "Selected Gate Image (Sum/Max)"=w263:T28, "Current Folder"=w278:path, "AlliGator IV DVR out"=w262:refnum<data-value>)  [unwired: 6 in]
      n82 = call "Show Animated Busy Icon with Message.vi"("Already active? (F)"=w257, "Message"=w275, "Error In"=w260, "Target VI Refnum"=w264) -> ("Error Out"=w274:errorcluster)  [unwired: 7 in]
      n83 = call "AlliGator Settings Storage.vi"("Get(F)/Set"=FALSE, "AlliGator Settings List"=AlliGator_Settings_List."Source Image:Intensity Threshold", "Error In"=w274) -> ("Error Out"=w268:errorcluster, "Variant Data out"=w271:variant)  [unwired: 7 in]
      n84 = call-poly "Variant to Data.vi"("Variant"=w271) -> ("Value"=w266:dbl)  [unwired: 8 in]
      n85 = call "Threshold Max Image to ROIs.vi"("Error In"=w268, "Threshold"=w266, "Image Refnum in"=w263) -> ("Error Out"=w269:errorcluster, "ROIs"=w270:T26[])  [unwired: 7 in]
      n86 = Format Into String(format string="Computing ROIs based on Min Intensity %#g:\n", w266) -> (resulting string=w265:string)  [unwired: 2 in, 1 out]
      n87 = call "AlliGator Add Multiple Source Image ROIs.vi"("Header message"=w265, "Error In"=w269, "ROIs"=w270, "ROI Mask Image Path"=w278) -> ("Error Out"=w277:errorcluster, "Message"=w258:string)  [unwired: 6 in]
      n88 = call "Hide Animated Busy Icon with Message.vi"("Already active? (F)"=w257, "Error In"=w277, "Target VI reference"=w264) -> ("Error Out"=w276:errorcluster)  [unwired: 8 in]
    }
    frame "Image:Create ROI(s) from Pixels with Peak above Min_Scriptable" {
      w283 = FALSE  # Max
      # "\"Create ROI from Pixels with Peak above Min\""
      n89 = call "AlliGator IV Selected Max or Sum Image.vi"("Sum (T)/ Max (F)"=w283, "AlliGator IV DVR in"=w287) -> ("Selected Gate Image (Sum/Max)"=w284:T28, "Current Folder"=w286:path, "AlliGator IV DVR out"=w285:refnum<data-value>)  [unwired: 6 in, 1 out]
      n90 = call "Show Animated Busy Icon with Message.vi"("Already active? (F)"=w281, "Message"=w298, "Target VI Refnum"=w288) -> ("Error Out"=w301:errorcluster)  [unwired: 8 in]
      n91 = call "AlliGator Settings Storage.vi"("Get(F)/Set"=FALSE, "AlliGator Settings List"=AlliGator_Settings_List."Source Image:Peak Threshold", "Error In"=w301) -> ("Error Out"=w292:errorcluster, "Variant Data out"=w295:variant)  [unwired: 7 in]
      n92 = call-poly "Variant to Data.vi"("Variant"=w295) -> ("Value"=w290:dbl)  [unwired: 8 in]
      n93 = call "Threshold Max Image to ROIs.vi"("Error In"=w292, "Threshold"=w290, "Image Refnum in"=w284) -> ("Error Out"=w293:errorcluster, "ROIs"=w294:T26[])  [unwired: 7 in]
      n94 = Format Into String(format string="Computing ROIs based on Min Peak Value %#g:\n", w290) -> (resulting string=w289:string)  [unwired: 2 in, 1 out]
      n95 = call "AlliGator Add Multiple Source Image ROIs.vi"("Header message"=w289, "Error In"=w293, "ROIs"=w294, "ROI Mask Image Path"=w286) -> ("Error Out"=w300:errorcluster, "Message"=w282:string)  [unwired: 6 in]
      n96 = call "Hide Animated Busy Icon with Message.vi"("Already active? (F)"=w281, "Error In"=w300, "Target VI reference"=w288) -> ("Error Out"=w299:errorcluster)  [unwired: 8 in]
    }
    frame "Image:Delete All ROIs" {
      # "\"Image:Delete All ROIs\""
      n97 = Bundle By Name(cluster=T6 {"AlliGator Q Event"=enum."Image:Source Image ROI Storage", "Data"=variant} ("Alligator Atomic Action"), "Data"=AlliGator_ROI_Manager_Actions."Delete All ROIs" ("Action")) -> (w306:T6)
      n98 = call-poly "AlliGator Add Action(s) to Stack.vi"("Elements Order in Action Stack (Default: 2 BEFORE 1)"=Alligator_Elements_Order_in_Action_Stack."Enqueue 2 BEFORE 1", "Error In"=w304, "Alligator Atomic Action"=w306, "Alligator Queue Element 1"=w312) -> ("Error Out"=w303:errorcluster, "Alligator Queue Element 1 (+ 2)"=w309:T6[])  [unwired: 6 in]
    }
    frame "Image:Delete All Unselected ROIs" {
      # "\"Image:Delete All Unselected ROIs\""
      n99 = Bundle By Name(cluster=T6 {"AlliGator Q Event"=enum."Image:Source Image ROI Storage", "Data"=variant} ("Alligator Atomic Action"), "Data"=AlliGator_ROI_Manager_Actions."Delete All Unselected ROIs" ("Action")) -> (w316:T6)
      n100 = call-poly "AlliGator Add Action(s) to Stack.vi"("Elements Order in Action Stack (Default: 2 BEFORE 1)"=Alligator_Elements_Order_in_Action_Stack."Enqueue 2 BEFORE 1", "Error In"=w314, "Alligator Atomic Action"=w316, "Alligator Queue Element 1"=w322) -> ("Error Out"=w313:errorcluster, "Alligator Queue Element 1 (+ 2)"=w319:T6[])  [unwired: 6 in]
    }
    frame "Image:Delete Existing ROIs Option" {
      # "\"Image:Delete Existing ROIs Option\""
      n101 = call "AlliGator skippable_Delete Existing ROIs Dialog Window.vi"("Error In"=w324) -> ("Error Out"=w327:errorcluster, "Delete"=w326:bool)  [unwired: 9 in]
      n102 = case shown="True" w326 {
        tunnel: w327 -> [w331 w336]
        tunnel: [w331 w334] -> w325
        tunnel: [_ w333] -> w323
        frame False {
        }
        frame True {
          n103 = call-poly "AlliGator Source Image ROI Storage [PM].vi"("Error In"=w336, "Current ROI Descriptor"=T26 {"Global Rectangle"=[], "Contours"=[]}, "Action"=AlliGator_ROI_Manager_Actions."Delete All ROIs") -> ("Error Out"=w334:errorcluster, "Message"=w333:string)  [unwired: 2 in, 5 out]
        }
      }
    }
    frame "Image:Delete ROI" {
      # "\"Image:Delete ROI\""
      n104 = Bundle By Name(cluster=T6 {"AlliGator Q Event"=enum."Image:Source Image ROI Storage", "Data"=variant} ("Alligator Atomic Action"), "Data"=AlliGator_ROI_Manager_Actions."Delete Current ROI" ("Action")) -> (w340:T6)
      n105 = call-poly "AlliGator Add Action(s) to Stack.vi"("Elements Order in Action Stack (Default: 2 BEFORE 1)"=Alligator_Elements_Order_in_Action_Stack."Enqueue 2 BEFORE 1", "Error In"=w338, "Alligator Atomic Action"=w340, "Alligator Queue Element 1"=w346) -> ("Error Out"=w337:errorcluster, "Alligator Queue Element 1 (+ 2)"=w343:T6[])  [unwired: 6 in]
    }
    frame "Image:Delete ROI(s) based on ROI Characteristics" {
      n106 = call "AlliGator Get Selected Image to Display.vi"("Error In"=w354, "AlliGator IV DVR in"=w358) -> ("Error Out"=w359:errorcluster, "Image out"=w355:T28, "AlliGator IV DVR out"=w357:refnum<data-value>, "ROI Mask"=w351:T28)  [unwired: 4 in, 2 out]
      n107 = call "Show Animated Busy Icon with Message.vi"("Already active? (F)"=w347, "Message"=w352, "Error In"=w359, "Target VI Refnum"=w348) -> ("Error Out"=w356:errorcluster)  [unwired: 7 in]
      n108 = case shown="No Error" w356 {
        selector: w356 -> [w365 w366]
        tunnel: w355 -> [w364 _]
        tunnel: w351 -> [w363 _]
        tunnel: [w362 _] -> w353
        tunnel: [w361 w366] -> w350
        frame No Error {
          n109 = call "AlliGator Reject Source Image ROIs based on Characteristics.vi"("error in (no error)"=w365, "ROI Mask Refnum"=w363, "Source Image Refnum"=w364) -> ("error out"=w361:errorcluster, "ROI Characteristics String"=w362:string)  [unwired: 7 in]
        }
        frame Error {
        }
      }
      n110 = call "Hide Animated Busy Icon with Message.vi"("Already active? (F)"=w347, "Error In"=w350, "Target VI reference"=w348) -> ("Error Out"=w349:errorcluster)  [unwired: 8 in]
    }
    frame "Image:Export ROI Description to Notebook" {
      # "\"Export ROI Description to Notebook\""
      n111 = Variant To Data(type=T27 {"Image Control Label"="", "ROI Descriptor"={"Global Rectangle"=[], "Contours"=[]}} ("cluster"), Variant=w387) -> (data=w375:T27, error out=w377:errorcluster)  [unwired: 1 in]
      n112 = case shown="No Error" w377 {
        selector: w377 -> [w389 _]
        tunnel: [w391 w394] -> w383
        tunnel: w375 -> [w390 w395]
        tunnel: w376 -> [_ w398]
        tunnel: [w390 w396] -> w374
        tunnel: [w389 w392] -> w373
        frame No Error {
          n113 = Unbundle By Name(w390) -> ("ROI Descriptor"=w391:T26)
        }
        frame Error {
          n114 = Unbundle By Name(w398) -> ("Registered Events Ctrl Refnums.Source Image Display"=w397:refnum<vi>)
          n115 = property class="ImageControl"(reference=w397) -> (error out=w392:errorcluster, "ROI"=w394:T72)  [unwired: 1 in, 1 out]
          n116 = Bundle By Name(cluster=w395, "ROI Descriptor"=w394, "Image Control Label"="Source Image") -> (w396:T27)
        }
      }
      n117 = call "Show Animated Busy Icon with Message.vi"("Already active? (F)"=w368, "Message"=w371, "Error In"=w373, "Target VI Refnum"=w369) -> ("Error Out"=w372:errorcluster)  [unwired: 7 in]
      n118 = call "Get ROI Area.vi"("Error In"=w372, "ROI Descriptor"=w383) -> ("Error Out"=w382:errorcluster, "Number of Pixels"=w381:u32)  [unwired: 8 in]
      n119 = call "AlliGator Find ROI Name.vi"("Error In"=w382, "ROI Descriptor"=w374) -> ("Error Out"=w385:errorcluster, "Image Control ROI Description"=w384:T73)  [unwired: 7 in, 1 out]
      n120 = call "AlliGator Format ROI Description for Notebook.vi"("error in (no error)"=w385, "# Pixels"=w381, "ROI Descriptor"=w384) -> ("error out"=w380:errorcluster, "Message"=w378:string)  [unwired: 7 in]
      n121 = call "Hide Animated Busy Icon with Message.vi"("Already active? (F)"=w368, "Error In"=w380, "Target VI reference"=w369) -> ("Error Out"=w370:errorcluster)  [unwired: 8 in]
    }
    frame "Image:Identify ROIs in Mask Image" {
      # "\"Identify ROIs in Mask Image\""
      n122 = call-poly "Variant to Data.vi"("Variant"=w407) -> ("String"=w406:string)  [unwired: 8 in]
      n123 = call "Show Animated Busy Icon with Message.vi"("Already active? (F)"=w399, "Message"=w402, "Error In"=w404, "Target VI Refnum"=w400) -> ("Error Out"=w403:errorcluster)  [unwired: 7 in]
      n124 = call "AlliGator Mask Image to ROIs.vi"("error in"=w403, "Mask Image Name (Default: none)"=w406, "Data Value Reference in"=w409) -> ("error out"=w410:errorcluster, "Message"=w405:string, "Data Value Reference out"=w408:refnum<data-value>)  [unwired: 6 in]
      n125 = call "Hide Animated Busy Icon with Message.vi"("Already active? (F)"=w399, "Error In"=w410, "Target VI reference"=w400) -> ("Error Out"=w401:errorcluster)  [unwired: 8 in]
    }
    frame "Image:Image Contrast" {
      w433 = -1074396120  # Not an image
      # "\"Image Contrast\""
      n126 = Variant To Data(type=T28 refnum ("Image out"), Variant=w416) -> (data=w414:T28, error out=w415:errorcluster)  [unwired: 1 in]
      n127 = call "Show Animated Busy Icon with Message.vi"("Already active? (F)"=w421, "Message"=w427, "Target VI Refnum"=w428) -> ("Error Out"=w437:errorcluster)  [unwired: 8 in]
      n128 = Unbundle By Name(w429) -> ("Dataset Control Refnums.Image Color Scale"=w430:refnum<vi>, "Registered Events Ctrl Refnums.Source Image Display"=w419:refnum<vi>, "Image Histogram Ctrl Refnums.Image Histogram"=w418:refnum<vi>)
      n129 = call "AlliGator Get Selected Image to Display.vi"("Error In"=w437, "AlliGator IV DVR in"=w426) -> ("Error Out"=w424:errorcluster, 1:"Displayed Image"=w431:T28, "Image out"=w413:T28, "AlliGator IV DVR out"=w425:refnum<data-value>, 4:"Displayed Image"=w423:T40)  [unwired: 4 in, 1 out]
      n130 = call "Alligator Variables Storage.vi"("Get(F)/Set"=FALSE, "AlliGator Variable"=AlliGator_Variables_List."X_Source Image:Palette Information" ("Alligator Variable"), "Error In"=w424) -> ("Error Out"=w436:errorcluster, "Data out"=w442:variant)  [unwired: 6 in, 1 out]
      n131 = Select(t=w413, s=w415, f=w414) -> (s? t:f=w412:T28)
      n132 = Variant To Data(error in=w436, type=T19 {"Palette Name [# Colors,int?,inv?]"="", "Palette Type"=0, "Palette Colors"=[], "Interpolate?"=FALSE} ("Image Display Palette Information"), Variant=w442) -> (data=w439:T19, error out=w434:errorcluster)
      n133 = call "AlliGator Set Image Display Range.vi"("Display Image Control Refnum"=w419, "Image Histogram"=w418, "Error In"=w424, "Displayed Image?"=w423, "Displayed Image"=w431, "Image to Display"=w412) -> ("Error Out"=w443:errorcluster, "Palette Display Range"=w440:cluster{"Min Value":dbl, "Max Value":dbl}, "Image Display Range"=w420:cluster{"Min Value":dbl, "Max Value":dbl})  [unwired: 2 in, 1 out]
      n134 = Merge Errors(w443, w434) -> (w435:errorcluster)
      n135 = case shown="\"Single Gate\", Default" w423 {
        tunnel: w435 -> [w457 w458]
        tunnel: w440 -> [w449 _]
        tunnel: w439 -> [w454 _]
        tunnel: w430 -> [w456 _]
        tunnel: w419 -> [w455 _]
        tunnel: [w453 w458] -> w422
        tunnel: w420 -> [w450 _]
        frame "Single Gate", Default {
          n136 = property on="Property Node" class="ColRmp (strict)"(reference=w456) -> (reference out=w451:refnum<vi>, "Scale.High Color"=w447:u32, "Scale.Low Color"=w448:u32)  [unwired: 1 in, 1 out]
          n137 = call "Image Display Set Color Palette.vi"("Image High Color"=w447, "Image Low Color"=w448, "Error In"=w457, "Image Display Range"=w450, "Image Display Palette Information"=w454, "Display Image Control Refnum"=w455) -> ("Error Out"=w452:errorcluster)  [unwired: 5 in]
          n138 = call "Set Color Ramp Palette v3.vi"("Image High Color"=w447, "Image Low Color"=w448, "error in (no error)"=w452, "Image Display Range"=w449, "Image Display Palette Information"=w454, "ColorRamp in"=w451) -> ("Error Out"=w453:errorcluster)  [unwired: 3 in, 2 out]
        }
        frame "Mask Image" {
        }
      }
      n139 = call "Hide Animated Busy Icon with Message.vi"("Already active? (F)"=w421, "Error In"=w422, "Target VI reference"=w428) -> ("Error Out"=w432:errorcluster)  [unwired: 8 in]
      n140 = call <vilib>:"Clear Errors.vi"("error in (no error)"=w432, "specific error code to clear (0: all)"=w433) -> ("error out"=w445:errorcluster)  [unwired: 4 in, 1 out]
    }
    frame "Image:Image Histogram Cursor Move" {
      n141 = Bundle By Name(cluster=T6 {"AlliGator Q Event"=enum."Image:Set Image Histogram Cursor Move Flag", "Data"=variant} ("element"), "Data"=FALSE) -> (w460:T6)
      n142 = Build Array (concatenate)(T6[] [{"AlliGator Q Event"=enum."Image:Image Histogram", "Data"=variant}, {"AlliGator Q Event"=enum."Image:Image Contrast", "Data"=variant}] ("element"), w460) -> (w462:T6[])
      n143 = call-poly "AlliGator Add Action(s) to Stack.vi"("Elements Order in Action Stack (Default: 2 BEFORE 1)"=Alligator_Elements_Order_in_Action_Stack."Enqueue 2 BEFORE 1", "Alligator Queue Element 2"=w462, "Alligator Queue Element 1"=w466) -> ("Alligator Queue Element 1 (+ 2)"=w464:T6[])  [unwired: 7 in, 1 out]
    }
    frame "Image:Image Histogram" {
      # "\"Image Histogram\""
      n144 = Unbundle By Name(w475) -> ("Image Histogram Ctrl Refnums.Image Histogram Active"=w476:refnum<vi>)
      n145 = property on="Property Node" class="Bool (strict)"(reference=w476) -> ("Value"=w474:bool)  [unwired: 1 in, 2 out]
      n146 = case shown="True" w474 {
        tunnel: w479 -> [_ w501]
        tunnel: w478 -> [_ w497]
        tunnel: [_ w503] -> w477
        tunnel: w475 -> [_ w502]
        tunnel: w473 -> [_ w498]
        tunnel: w472 -> [w481 w500]
        tunnel: [w481 w499] -> w471
        tunnel: w470 -> [_ w486]
        frame False {
        }
        frame True {
          n147 = Variant To Data(type=T28 refnum ("Image out"), Variant=w486) -> (data=w483:T28, error out=w484:errorcluster)  [unwired: 1 in]
          n148 = call "Show Animated Busy Icon with Message.vi"("Already active? (F)"=w497, "Message"=w498, "Target VI Refnum"=w501) -> ("Error Out"=w496:errorcluster)  [unwired: 8 in]
          n149 = Unbundle By Name(w502) -> ("Dataset Control Refnums.Gate Image Slide"=w487:refnum<vi>, "Image Histogram Ctrl Refnums"=w494:T14, "Dataset Control Refnums.Displayed Image"=w482:refnum<vi>)
          n150 = case shown="Error .." w484 {
            tunnel: w500 -> [w508 w514]
            tunnel: [w508 w513] -> w499
            tunnel: w496 -> [w506 w512]
            tunnel: [w507 w511] -> w493
            tunnel: [w506 w510] -> w491
            tunnel: [w504 w509] -> w490
            tunnel: w483 -> [w507 _]
            tunnel: w482 -> [w505 _]
            frame No Error {
              n151 = property class="Enum (strict)"(reference=w505) -> ("Value"=w504:T40)  [unwired: 1 in, 2 out]
            }
            frame Error {
              n152 = call "AlliGator Get Selected Image to Display.vi"("Error In"=w512, "AlliGator IV DVR in"=w514) -> ("Error Out"=w510:errorcluster, "Image out"=w511:T28, "AlliGator IV DVR out"=w513:refnum<data-value>, "Displayed Image"=w509:T40)  [unwired: 4 in, 2 out]
            }
          }
          n153 = case shown="\"Sum of All Gates\", Default" w490 {
            selector: w490 -> [w517 w520]
            tunnel: [TRUE ("Visible") _] -> w492
            tunnel: [w517 w520] -> w489
            tunnel: w487 -> [w516 _]
            tunnel: [w515 u16 0 ("Value")] -> w488
            frame "Single Gate" {
              n154 = property on="Property Node" class="Slide (strict)"(reference=w516) -> ("Value"=w515:u16)  [unwired: 1 in, 2 out]
            }
            frame "Sum of All Gates", Default {
            }
          }
          n155 = property on="Property Node" class="Slide (strict)"(reference=w487, "Visible"=w492) -> ()  [unwired: 1 in, 2 out]
          n156 = call "AlliGator Single Image Histogram.vi"("Gate Slider"=w488, "Error In"=w491, "Displayed Image"=w489, "Image Histogram Ctrl Refnums"=w494, "Image in"=w493) -> ("Error Out"=w495:errorcluster)  [unwired: 3 in, 3 out]
          n157 = call "Hide Animated Busy Icon with Message.vi"("Already active? (F)"=w497, "Error In"=w495, "Target VI reference"=w501) -> ("Error Out"=w503:errorcluster)  [unwired: 8 in]
        }
      }
    }
    frame "Image:Load ROI" {
      # "\"Load ROI\""
      n158 = Variant To Data(error in=w522, type=refnum<vi> refnum ("CtlRef"), Variant=w534) -> (data=w532:refnum<vi>, error out=w531:errorcluster)
      n159 = call "Show Animated Busy Icon with Message.vi"("Already active? (F)"=w523, "Message"=w521, "Error In"=w531, "Target VI Refnum"=w526) -> ("Error Out"=w529:errorcluster)  [unwired: 7 in]
      n160 = call "AlliGator Load ROI v3.vi"("Error In"=w529, "Dialog (T)"=TRUE, "Source Image Refnum"=w532) -> ("Error Out"=w530:errorcluster, "Message"=w524:string)  [unwired: 2 in, 5 out]
      n161 = call "Hide Animated Busy Icon with Message.vi"("Already active? (F)"=w523, "Error In"=w530, "Target VI reference"=w526) -> ("Error Out"=w528:errorcluster)  [unwired: 8 in]
    }
    frame "Image:Merge All ROIs" {
      # "\"Image:Merge All ROIs\""
      n162 = Bundle By Name(cluster=T6 {"AlliGator Q Event"=enum."Image:Source Image ROI Storage", "Data"=variant} ("Alligator Atomic Action"), "Data"=AlliGator_ROI_Manager_Actions."Merge All ROIs" ("Action")) -> (w539:T6)
      n163 = call-poly "AlliGator Add Action(s) to Stack.vi"("Elements Order in Action Stack (Default: 2 BEFORE 1)"=Alligator_Elements_Order_in_Action_Stack."Enqueue 2 BEFORE 1", "Error In"=w537, "Alligator Atomic Action"=w539, "Alligator Queue Element 1"=w545) -> ("Error Out"=w536:errorcluster, "Alligator Queue Element 1 (+ 2)"=w542:T6[])  [unwired: 6 in]
    }
    frame "Image:Mouse Move" {
      # "\"Image:Mouse Move\""
      n164 = Variant To Data(error in=w546, Variant=w550) -> (data=w549:T74, error out=w548:errorcluster)  [unwired: 1 in]
      n165 = call "AlliGator Source Image Mouse Move Event.vi"("error in"=w548, "Image User Event Data"=w549, "AlliGator Events in"=w552) -> ("error out"=w547:errorcluster, "AlliGator Events out"=w551:T6[])  [unwired: 7 in]
    }
    frame "Image:Mouse Up" {
      # "\"Image:Mouse Up\""
      n166 = Unbundle By Name(w557) -> ("Dataset Control Refnums"=w556:T12)
      n167 = Variant To Data(error in=w563, Variant=w564) -> (data=w558:T76, error out=w559:errorcluster)  [unwired: 1 in]
      n168 = call "AlliGator Source Image Mouse Up Event.vi"("Dataset Ctrl Refnums"=w556, "error in (no error)"=w559, "Image Mouse Up Event Data"=w558, "AlliGator Actions in"=w562) -> ("error out"=w560:errorcluster, "AlliGator Actions out"=w561:T6[])  [unwired: 6 in]
    }
    frame "Image:Overlay ROI Median" {
      # "\"Image:Overlay ROI Median\""
      n169 = call "AlliGator Overlay ROI Median.vi"("AlliGator Ctrl Refnums"=w569, "error in (no error)"=w567, "AlliGator IV DVR in"=w571) -> ("error out"=w568:errorcluster, "AlliGator IV DVR out"=w570:refnum<data-value>)  [unwired: 7 in]
    }
    frame "Image:Paste ROI Definition" {
      # "\"Paste ROI Definition\""
      n170 = Unbundle By Name(w578) -> ("Registered Events Ctrl Refnums.Source Image Display"=w577:refnum<vi>)
      n171 = invoke on="Invoke Node" class="App" method="Clipboard.Read"() -> (error out=w584:errorcluster, "Read Clipbrd"=w585:string)  [unwired: 3 in, 1 out]
      n172 = call "ROI Description to ROI.vi"("error in (no error)"=w584, "ROI Description"=w585) -> ("error out"=w583:errorcluster, "Current ROI Descriptor(s)"=w582:T26)  [unwired: 8 in]
      n173 = disable-structure "Diagram Disable Structure" shown="Enabled" {
        disable-tunnel: w583 -> [w593 w594]
        disable-tunnel: w582 -> [w592 w595]
        disable-tunnel: [w590 w594] -> w581
        disable-tunnel: [w589 w595] -> w580
        disable-tunnel: [w588 _] -> w574
        frame Disabled {
          n174 = call-poly "AlliGator Source Image ROI Storage [PM].vi"("Error In"=w593, "Current ROI Descriptor"=w592, "Action"=AlliGator_ROI_Manager_Actions."Store New ROI" ("Enum")) -> ("Error Out"=w590:errorcluster, "Current ROI Descriptor"=w589:T26, "Message"=w588:string)  [unwired: 2 in, 4 out]
        }
        frame Enabled {
        }
      }
      n175 = call "Image Display Get-Set ROI.vi"("Get(F)/Set"=TRUE ("Get(F)/Set(T)"), "Error In"=w581, "ROI Descriptor in"=w580, "Image Display Refnum"=w577) -> ("Error Out"=w579:errorcluster)  [unwired: 3 in, 4 out]
    }
    frame "Image:Python Function Source Image Event" {
      # "\"Python Function Source Image Event\""
      n176 = Variant To Data(Variant=w613) -> (data=w612:T81, error out=w611:errorcluster)  [unwired: 2 in]
      n177 = call "Show Animated Busy Icon with Message.vi"("Already active? (F)"=w597, "Message"=w610, "Error In"=w611, "Target VI Refnum"=w609) -> ("Error Out"=w599:errorcluster)  [unwired: 7 in]
      n178 = call "AlliGator Image Python Function Handler Core.vi"("error in (no error)"=w599, "Data Value Reference in"=w602, "Image Event"=w612) -> ("error out"=w600:errorcluster, "Message"=w598:string, "Data Value Reference out"=w601:refnum<data-value>, "Alligator Atomic Action"=w603:T6[])  [unwired: 5 in]
      n179 = call "Hide Animated Busy Icon with Message.vi"("Already active? (F)"=w597, "Error In"=w600, "Target VI reference"=w609) -> ("Error Out"=w606:errorcluster)  [unwired: 8 in]
      n180 = call-poly "AlliGator Add Action(s) to Stack.vi"("Elements Order in Action Stack (Default: 2 BEFORE 1)"=Alligator_Elements_Order_in_Action_Stack."Enqueue 2 BEFORE 1", "Error In"=w606, "Alligator Queue Element 2"=w603, "Alligator Queue Element 1"=w608) -> ("Error Out"=w604:errorcluster, "Alligator Queue Element 1 (+ 2)"=w607:T6[])  [unwired: 6 in]
    }
    frame "Image:ROI to Individual Pixel ROIs" {
      w615 = FALSE ("Get (F)/ Set (T)")
      w620 = "Abort ROI Creation" ("Abort Button Name (Abort)")
      # "\"ROI to Individual Pixel ROIs\""
      n181 = Unbundle By Name(w633) -> ("Registered Events Ctrl Refnums.Source Image Display"=w635:refnum<vi>, "Other AlliGator Ctrl Refnums.Abort ROI Creation"=w627:refnum<vi>)
      n182 = call "AlliGator IV Type of Displayed Image.vi"("Get (F)/ Set (T)"=w615, "AlliGator IV DVR in"=w625) -> ("error out"=w617:errorcluster, "Type of Displayed Image"=w616:T40, "AlliGator IV DVR out"=w618:refnum<data-value>)  [unwired: 7 in]
      n183 = case shown="\"Mask Image\"" w616 {
        tunnel: [w646 w649 w655] -> w624
        tunnel: [w645 w650 w656] -> w623
        tunnel: [w644 w648 w654] -> w622
        tunnel: w618 -> [w642 w652 w658]
        tunnel: w617 -> [w641 w651 w657]
        tunnel: w615 -> [_ w647 w653]
        frame "Single Gate", Default {
          n184 = call "AlliGator IV Selected Max or Sum Image.vi"("Error In"=w641, "Sum (T)/ Max (F)"=FALSE, "AlliGator IV DVR in"=w642) -> ("Error Out"=w644:errorcluster, "Selected Gate Image (Sum/Max)"=w646:T28, "AlliGator IV DVR out"=w645:refnum<data-value>)  [unwired: 5 in, 1 out]
        }
        frame "White Ligth Image" {
          n185 = call "AlliGator IV White Light Image.vi"("Get (F)/ Set (T)"=w647, "error in (no error)"=w651, "AlliGator IV DVR in"=w652) -> ("error out"=w648:errorcluster, "White Light Image"=w649:T28, "AlliGator IV DVR out"=w650:refnum<data-value>)  [unwired: 6 in]
        }
        frame "Mask Image" {
          n186 = call "AlliGator IV Mask Image.vi"("Get (F)/ Set (T)"=w653, "error in (no error)"=w657, "AlliGator IV DVR in"=w658) -> ("error out"=w654:errorcluster, "Mask Image"=w655:T28, "AlliGator IV DVR out"=w656:refnum<data-value>)  [unwired: 6 in]
        }
      }
      n187 = call-poly "Variant to Data.vi"("Variant"=w630) -> ("Value"=w629:i32)  [unwired: 8 in]
      n188 = property on="Property Node" class="ImageControl"(reference=w635, error in=w622) -> (error out=w639:errorcluster, "ROI"=w638:T72)  [unwired: 1 out]
      n189 = call "Show Animated Busy Icon with Message.vi"("Animated Busy Icon Control Name (Animated Busy Icon)"=w620, "Already active? (F)"=w619, "Message"=w634, "Error In"=w639, "Target VI Refnum"=w628) -> ("Error Out"=w626:errorcluster)  [unwired: 6 in]
      n190 = call "IMAQ GetImageInfo"("Image"=w624) -> ("Y Resolution"=w636:i32, "X Resolution"=w637:i32)  [unwired: 3 in, 6 out]
      n191 = call "AlliGator Create Individual Pixel ROIs from ROI.vi"("Y Resolution"=w636, "X Resolution"=w637, "Error In"=w626, "Abort ROI Creation"=w627, "Selected ROI (-1: use ROI Descriptor)"=w629, "ROI"=w638) -> ("Error Out"=w631:errorcluster, "Message"=w621:string)  [unwired: 4 in]
      n192 = call "Hide Animated Busy Icon with Message.vi"("Animated Busy Icon Control Name (Animated Busy Icon)"=w620, "Already active? (F)"=w619, "Error In"=w631, "Target VI reference"=w628) -> ("Error Out"=w632:errorcluster)  [unwired: 7 in]
    }
    frame "Image:Save Displayed Image with Overlay" {
      # "\"Save Displayed Image with Overlay\""
      n193 = Unbundle By Name(w671) -> ("Registered Events Ctrl Refnums.Source Image Display"=w683:refnum<vi>, "Dataset Control Refnums.Gate Image Slide"=w670:refnum<vi>)
      n194 = call-poly "Variant to Data.vi"("Variant"=w681) -> ("Value"=w677:bool)  [unwired: 8 in]
      n195 = call "AlliGator Get Image File Format.vi"() -> ("error out"=w676:errorcluster, "Transparent Mask Color"=w659:u32, "File Extension (.xxx)"=w673:string, "Image File Format"=w679:T29)  [unwired: 8 in]
      n196 = call "Show Animated Busy Icon with Message.vi"("Already active? (F)"=w660, "Message"=w663, "Error In"=w676, "Target VI Refnum"=w661) -> ("Error Out"=w664:errorcluster)  [unwired: 7 in]
      n197 = call "AlliGator Build Saved Image Path.vi"("Gate Image Slide"=w670, "Error In"=w664, "File Extension"=w673, "AlliGator IV DVR in"=w668) -> ("Error Out"=w675:errorcluster, "appended path"=w674:path, "AlliGator IV DVR out"=w667:refnum<data-value>)  [unwired: 5 in]
      n198 = call "Image File Dialog (Optional).vi"("Dialog?"=w677, "Error In"=w675, "Image File Format in"=w679, "Default file path in"=w674) -> ("Error Out"=w672:errorcluster, "Image File Format out"=w678:T29, "file path out"=w680:path)  [unwired: 5 in]
      n199 = call "Image Display Save Image.vi"("Mask Color (Transparent)"=w659, "error in (no error)"=w672, "Saved Image File Format"=w678, "File Path in"=w680, "Display Image Control Refnum"=w683) -> ("Error Out"=w682:errorcluster, "File Path out"=w669:path)  [unwired: 5 in]
      n200 = call "Hide Animated Busy Icon with Message.vi"("Already active? (F)"=w660, "Error In"=w682, "Target VI reference"=w661) -> ("Error Out"=w662:errorcluster)  [unwired: 8 in]
      n201 = Format Into String(format string="Displayed source Image saved with overlay to %s", error in=w662, w669) -> (resulting string=w666:string, error out=w665:errorcluster)  [unwired: 1 in]
    }
    frame "Image:Save Image as Hot Pixel Mask" {
      # "\"Image:Save Image as Hot Pixel Mask\""
      n202 = in-place "In Place Element Structure" {
        in-place-border: [w728] -> w711
        in-place-border: [w727] -> w710
        in-place-border: [w726] -> w709
        in-place-border: [w724] -> w687
        n203 = in-place-dvr #5 ("Data Value Reference Read / Write Element")(w689) -> (w725:T34, w724:errorcluster)
        n204 = Unbundle By Name(w725) -> ("Single Data Point Path"=w728:path, "[Time-Series Paths]"=w727:path[], "Current Dataset"=w726:i32)
        n205 = in-place-dvr #5 ("Data Value Reference Read / Write Element")() -> (w688:refnum<data-value>)  [unwired: 1 in, 1 out]
      }
      n206 = Unbundle By Name(w715) -> ("Registered Events Ctrl Refnums.Source Image Display"=w701:refnum<vi>)
      n207 = Variant To Data(type=w701, Variant=w702) -> (data=w696:refnum<vi>, error out=w695:errorcluster)  [unwired: 1 in]
      n208 = property on="Property Node" class="ImageControl"(reference=w696, error in=w695) -> (error out=w693:errorcluster, "Value"=w694:variant)  [unwired: 1 out]
      n209 = Variant To Data(error in=w693, Variant=w694) -> (data=w692:T28, error out=w691:errorcluster)  [unwired: 1 in]
      n210 = call "AlliGator Get Destination Folder.vi"("Current Data Set (-1: single)"=w709, "Time-Series Paths"=w710, "Single Data Point Path"=w711) -> ("Data Point Name"=w690:string, "Destination Folder path"=w721:path)  [unwired: 5 in, 2 out]
      n211 = Merge Errors(w691, w687) -> (w700:errorcluster)
      n212 = call "Show Animated Busy Icon with Message.vi"("Already active? (F)"=w703, "Message"=w705, "Error In"=w700, "Target VI Refnum"=w704) -> ("Error Out"=w706:errorcluster)  [unwired: 7 in]
      n213 = Concatenate Strings(w690, " Hot Pixel Mask" ("string"), ".PNG" ("string")) -> (w716:string)
      n214 = Build Path(base path=w721, name or relative path=w716) -> (appended path=w720:path)
      n215 = call "Image File Dialog (Optional).vi"("Dialog?"=TRUE, "Error In"=w706, "Image File Format in"=Image_Save_File_Format."PNG", "Default file path in"=w720) -> ("Error Out"=w717:errorcluster, "Image File Format out"=w718:T29, "file path out"=w719:path)  [unwired: 5 in]
      n216 = call "AlliGator Save Hot Pixel Mask Image.vi"("error in (no error)"=w717, "Saved Image File Format"=w718, "File Path in"=w719, "Image Refnum in"=w692) -> ("Error Out"=w707:errorcluster, "File Path out"=w712:path)  [unwired: 6 in]
      n217 = call "Hide Animated Busy Icon with Message.vi"("Already active? (F)"=w703, "Error In"=w707, "Target VI reference"=w704) -> ("Error Out"=w686:errorcluster)  [unwired: 8 in]
      n218 = Format Into String(format string="Hot Pixel Mask Image saved to %s", error in=w686, w712) -> (resulting string=w708:string, error out=w713:errorcluster)  [unwired: 1 in]
    }
    frame "Image:Save Image Data as TIFF" {
      # "\"Save Image Data as TIFF\""
      n219 = in-place "In Place Element Structure" {
        in-place-border: [w755] -> w737
        in-place-border: [w754] -> w736
        in-place-border: [w753] -> w735
        in-place-border: [w752] -> w734
        in-place-border: [w751] -> w733
        n220 = in-place-dvr #6 ("Data Value Reference Read / Write Element")(w730) -> (w750:T34)  [unwired: 1 out]
        n221 = Unbundle By Name(w750) -> ("Type of Displayed Image"=w755:T40, "Gate Image Slide"=w751:u16, "Single Data Point Path"=w752:path, "Phasor Plot Image"=w753:T28, "Displayed Image"=w754:T28)
        n222 = in-place-dvr #6 ("Data Value Reference Read / Write Element")() -> (w729:refnum<data-value>)  [unwired: 1 in, 1 out]
      }
      n223 = call-poly "Variant to Data.vi"("Variant"=w746) -> ("Value"=w744:bool)  [unwired: 8 in]
      n224 = case shown="True" w744 {
        tunnel: w737 -> [w758 _]
        tunnel: [w757 AlliGator_Saved_TIFF_Image_Type."Phasor" ("Displayed Image")] -> w743
        tunnel: [w756 _] -> w740
        frame False {
          n225 = case shown="\"-\"" w758 {
            tunnel: [_ AlliGator_Saved_TIFF_Image_Type."Single Gate" ("Displayed Image") AlliGator_Saved_TIFF_Image_Type."Sum of All Gates" ("Displayed Image")] -> w757
            tunnel: [w759 _ _] -> w756
            frame "-" {
              n226 = xnode ("Error Ring")() -> ("error out"=w759:errorcluster)
            }
            frame "Single Gate", Default {
            }
            frame "Sum of All Gates" {
            }
          }
        }
        frame True {
        }
      }
      n227 = Select(t=w735, s=w744, f=w736) -> (s? t:f=w745:T28)
      n228 = call "Show Animated Busy Icon with Message.vi"("Already active? (F)"=w731, "Message"=w738, "Error In"=w740, "Target VI Refnum"=w739) -> ("Error Out"=w748:errorcluster)  [unwired: 7 in]
      n229 = call "AlliGator Save Image Data to File.vi"("Time Gate"=w733, "error in (no error)"=w748, "Saved TIFF Image"=w743, "Image"=w745, "File Path in"=w734) -> ("error out"=w741:errorcluster, "Output String"=w742:string, "Message"=w732:string)  [unwired: 3 in, 1 out]
      n230 = call "Hide Animated Busy Icon with Message.vi"("Already active? (F)"=w731, "Message"=w742, "Error In"=w741, "Target VI reference"=w739) -> ("Error Out"=w747:errorcluster)  [unwired: 7 in]
    }
    frame "Image:Save Image Overlay Only" {
      # "\"Save Image Overlay Only\""
      n231 = Unbundle By Name(w783) -> ("Registered Events Ctrl Refnums.Source Image Display"=w794:refnum<vi>)
      n232 = in-place "In Place Element Structure" {
        in-place-border: [w806] -> w779
        in-place-border: [w805] -> w778
        in-place-border: [w804] -> w777
        in-place-border: [w802] -> w769
        n233 = in-place-dvr #7 ("Data Value Reference Read / Write Element")(w770) -> (w803:T34, w802:errorcluster)
        n234 = Unbundle By Name(w803) -> ("Single Data Point Path"=w806:path, "[Time-Series Paths]"=w805:path[], "Current Dataset"=w804:i32)
        n235 = in-place-dvr #7 ("Data Value Reference Read / Write Element")() -> (w767:refnum<data-value>)  [unwired: 1 in, 1 out]
      }
      n236 = call-poly "Variant to Data.vi"("Variant"=w786) -> ("Value"=w785:bool)  [unwired: 8 in]
      n237 = property on="Property Node" class="ImageControl"(reference=w794, error in=w769) -> (reference out=w795:refnum<vi>, error out=w793:errorcluster, "Label.Text"=w800:string)
      n238 = call "AlliGator Get Destination Folder.vi"("Current Data Set (-1: single)"=w777, "Time-Series Paths"=w778, "Single Data Point Path"=w779) -> ("Data Point Name"=w797:string, "Destination Folder path"=w798:path)  [unwired: 5 in, 2 out]
      n239 = call "AlliGator Get Image File Format.vi"("Error In"=w793) -> ("error out"=w791:errorcluster, "File Extension (.xxx)"=w796:string, "Image File Format"=w792:T29)  [unwired: 7 in, 1 out]
      n240 = call "Show Animated Busy Icon with Message.vi"("Already active? (F)"=w771, "Message"=w773, "Error In"=w791, "Target VI Refnum"=w772) -> ("Error Out"=w774:errorcluster)  [unwired: 7 in]
      n241 = Concatenate Strings(w800, " Overlay " ("string"), w797, w796) -> (w784:string)
      n242 = Build Path(base path=w798, name or relative path=w784) -> (appended path=w790:path)
      n243 = call "Image File Dialog (Optional).vi"("Dialog?"=w785, "Error In"=w774, "Image File Format in"=w792, "Default file path in"=w790) -> ("Error Out"=w787:errorcluster, "Image File Format out"=w788:T29, "file path out"=w789:path)  [unwired: 5 in]
      n244 = call "Image Display Save Overlay.vi"("error in (no error)"=w787, "Saved Image File Format"=w788, "File Path in"=w789, "Display Image Control Refnum"=w795) -> ("Error Out"=w775:errorcluster, "File Path out"=w780:path)  [unwired: 6 in]
      n245 = call "Hide Animated Busy Icon with Message.vi"("Already active? (F)"=w771, "Error In"=w775, "Target VI reference"=w772) -> ("Error Out"=w768:errorcluster)  [unwired: 8 in]
      n246 = Format Into String(format string="Image overlay saved to %s", error in=w768, w780) -> (resulting string=w776:string, error out=w781:errorcluster)  [unwired: 1 in]
    }
    frame "Image:Save ROI" {
      # "\"Save ROI\""
      n247 = Unbundle By Name(w813) -> ("Dataset Control Refnums.Current Data"=w812:refnum<vi>)
      n248 = Variant To Data(error in=w810, type=T31 {"Image Ctrl Ref"=refnum, "All ROIs?"=TRUE} ("Selected ROI"), Variant=w828) -> (data=w826:T31, error out=w809:errorcluster)
      n249 = Unbundle By Name(w826) -> ("Image Ctrl Ref"=w825:T32, "All ROIs?"=w823:bool)
      n250 = property on="Property Node" class="Str"(reference=w812, error in=w809) -> (error out=w808:errorcluster, "Value"=w811:string)  [unwired: 1 out]
      n251 = property on="Property Node" class="ImageControl"(reference=w825, error in=w808) -> (error out=w807:errorcluster, "Label.Text"=w824:string, "ROI"=w822:T72)  [unwired: 1 out]
      n252 = call "Show Animated Busy Icon with Message.vi"("Already active? (F)"=w814, "Message"=w817, "Error In"=w807, "Target VI Refnum"=w815) -> ("Error Out"=w818:errorcluster)  [unwired: 7 in]
      n253 = call "AlliGator Save ROI(s).vi"("Current Dataset Name"=w811, "Error In"=w818, "ROI Descriptor"=w822, "All ROIs?"=w823, "Image Label"=w824) -> ("Error Out"=w821:errorcluster, "Message"=w819:string)  [unwired: 5 in]
      n254 = call "Hide Animated Busy Icon with Message.vi"("Already active? (F)"=w814, "Error In"=w821, "Target VI reference"=w815) -> ("Error Out"=w816:errorcluster)  [unwired: 8 in]
    }
    frame "Image:Set Image Histogram Cursor Move Flag" {
      # "\"Image:Set Image Histogram Cursor Move Flag\""
      n255 = call-poly "Variant to Data.vi"("Variant"=w832) -> ("Value"=w831:bool)  [unwired: 8 in]
      n256 = call "AlliGator Image Contrast Status.vi"("Flag (in)"=w831, "Read/Write"=Read-Write."Write") -> ()  [unwired: 7 in, 1 out]
    }
    frame "Image:Set ROI Diameter" {
      # "\"Set ROI Diameter\""
      n257 = Unbundle By Name(w839) -> ("Registered Events Ctrl Refnums.Source Image Display"=w843:refnum<vi>)
      n258 = call "AlliGator Settings Storage.vi"("AlliGator Settings List"=AlliGator_Settings_List."Source Image:ROI Diameter") -> ("Error Out"=w842:errorcluster, "Variant Data out"=w846:variant)  [unwired: 9 in]
      n259 = call-poly "Variant to Data.vi"("Variant"=w846) -> ("Value"=w845:i32)  [unwired: 8 in]
      n260 = call "Image Display Set ROI Diameter.vi"("Error In"=w842, "ROI Diameter"=w845, "Display Image Control Refnum"=w843) -> ("Error Out"=w841:errorcluster)  [unwired: 8 in]
      n261 = Format Into String(format string=": %d", error in=w841, w845) -> (resulting string=w837:string, error out=w840:errorcluster)  [unwired: 1 in]
    }
    frame "Image:Set Source Image Mouse Move Flag" {
      # "\"Image:Set Source Image Mouse Move Flag\""
      n262 = call-poly "Variant to Data.vi"("Variant"=w854) -> ("Value"=w853:bool)  [unwired: 8 in]
      n263 = Unbundle By Name(w851) -> ("Registered Events Ctrl Refnums.Source Image Display"=w850:refnum<vi>)
      n264 = call "AlliGator Generic Image Display Mouse Move Flag.vi"("Image Control Refnum"=w850, "Flag (in)"=w853, "Read/Write"=Read-Write."Write") -> ()  [unwired: 6 in, 1 out]
    }
    frame "Image:Show Phasor Calibration Map ROI Centers" {
      # "\"Image:Show Phasor Calibration Map ROI Centers\""
      n265 = Unbundle By Name(w861) -> ("Registered Events Ctrl Refnums.Source Image Display"=w860:refnum<vi>, "Dataset Control Refnums.Source Image ROI Color"=w859:refnum<vi>)
      n266 = call "Show Animated Busy Icon with Message.vi"("Already active? (F)"=w867, "Message"=w866, "Target VI Refnum"=w868) -> ("Error Out"=w863:errorcluster)  [unwired: 8 in]
      n267 = call "AlliGator Show Phasor Calibration Map ROI Centers Overlay.vi"("Error In"=w863, "Source Image ROI Color"=w859, "Destination Image Control Refnum"=w860, "AlliGator IV DVR in"=w865) -> ("Error Out"=w862:errorcluster, "AlliGator IV DVR out"=w864:refnum<data-value>)  [unwired: 6 in]
      n268 = call "Hide Animated Busy Icon with Message.vi"("Already active? (F)"=w867, "Error In"=w862, "Target VI reference"=w868) -> ()  [unwired: 8 in, 1 out]
    }
    frame "Image:Source Image ROI Selection" {
      # "\"Source Image ROI Selection\""
      n269 = Variant To Data(Variant=w885) -> (data=w874:T82, error out=w884:errorcluster)  [unwired: 2 in]
      n270 = call "Show Animated Busy Icon with Message.vi"("Already active? (F)"=w880, "Error In"=w884, "Target VI Refnum"=w881) -> ("Error Out"=w882:errorcluster)  [unwired: 8 in]
      n271 = call "AlliGator Source Image Selection.vi"("AlliGator Ctrl Refnums"=w875, "error in (no error)"=w882, "ROI Selection Data"=w874) -> ("error out"=w873:errorcluster, "Alligator Queue Element out"=w878:T6[])  [unwired: 7 in]
      n272 = call "Hide Animated Busy Icon with Message.vi"("Already active? (F)"=w880, "Error In"=w873, "Target VI reference"=w881) -> ("Error Out"=w872:errorcluster)  [unwired: 8 in]
      n273 = call-poly "AlliGator Add Action(s) to Stack.vi"("Elements Order in Action Stack (Default: 2 BEFORE 1)"=Alligator_Elements_Order_in_Action_Stack."Enqueue 2 BEFORE 1", "Error In"=w872, "Alligator Queue Element 2"=w878, "Alligator Queue Element 1"=w879) -> ("Error Out"=w871:errorcluster, "Alligator Queue Element 1 (+ 2)"=w877:T6[])  [unwired: 6 in]
    }
    frame "Image:Source Image ROI Storage" {
      # "\"Source Image ROI Storage\""
      n274 = Variant To Data(type=AlliGator_ROI_Manager_Actions."Show All ROIs" ("Action"), Variant=w901) -> (data=w900:T25, error out=w893:errorcluster)  [unwired: 1 in]
      n275 = Unbundle By Name(w897) -> ("Registered Events Ctrl Refnums.Source Image Display"=w894:refnum<vi>)
      n276 = call "Image Display Get-Set ROI.vi"("Get(F)/Set"=FALSE ("Get(F)/Set(T)"), "Error In"=w893, "Image Display Refnum"=w894) -> ("Error Out"=w891:errorcluster, "ROI Descriptor out"=w888:T26, "Image Display Refnum (dup)"=w892:T32)  [unwired: 4 in, 2 out]
      n277 = call "ROI to Default ROI Name.vi"("Error In"=w891, "ROI"=w888) -> ("Error Out"=w903:errorcluster, "ROI Type String"=w902:string)  [unwired: 8 in]
      n278 = call-poly "AlliGator Source Image ROI Storage [PM].vi"("Error In"=w903, "Current ROI Descriptor"=w888, "Default Name (\"ROI\")"=w902, "Action"=w900) -> ("Error Out"=w898:errorcluster, "Current ROI Descriptor"=w896:T26, "Message"=w886:string)  [unwired: 1 in, 4 out]
      n279 = call "Image Display Get-Set ROI.vi"("Get(F)/Set"=TRUE ("Get(F)/Set(T)"), "Error In"=w898, "ROI Descriptor in"=w896, "Image Display Refnum"=w892) -> ("Error Out"=w895:errorcluster)  [unwired: 3 in, 4 out]
    }
    frame "Image:Store ROI" {
      # "\"Image:Store ROI\""
      n280 = Bundle By Name(cluster=T6 {"AlliGator Q Event"=enum."Image:Source Image ROI Storage", "Data"=variant} ("Alligator Atomic Action"), "Data"=AlliGator_ROI_Manager_Actions."Store New ROI" ("Action")) -> (w909:T6)
      n281 = call-poly "AlliGator Add Action(s) to Stack.vi"("Elements Order in Action Stack (Default: 2 BEFORE 1)"=Alligator_Elements_Order_in_Action_Stack."Enqueue 2 BEFORE 1", "Error In"=w907, "Alligator Atomic Action"=w909, "Alligator Queue Element 1"=w915) -> ("Error Out"=w906:errorcluster, "Alligator Queue Element 1 (+ 2)"=w912:T6[])  [unwired: 6 in]
    }
    frame "Image:Update Image Profile Plots" {
      # "\"Update Image Profile Plots\""
      n282 = Unbundle By Name(w928) -> ("Registered Events Ctrl Refnums.Source Image Display"=w929:refnum<vi>, "Decay Fit Map Ctrl Refnums.Decay Fit Parameter"=w927:refnum<vi>)
      n283 = property on="Property Node" class="Enum (strict)"(reference=w927, error in=w921) -> (error out=w922:errorcluster, "Value"=w926:T83)  [unwired: 1 out]
      n284 = call "Show Animated Busy Icon with Message.vi"("Already active? (F)"=w916, "Message"=w918, "Error In"=w922, "Target VI Refnum"=w917) -> ("Error Out"=w920:errorcluster)  [unwired: 7 in]
      n285 = call "AlliGator Send Plots to Image Profile Window.vi"("Image Control Refnum"=w929, "error in (no error)"=w920, "Fit Parameter"=w926, "AlliGator IV DVR in"=w925) -> ("error out"=w923:errorcluster, "AlliGator IV DVR out"=w924:refnum<data-value>)  [unwired: 6 in]
      n286 = call "Hide Animated Busy Icon with Message.vi"("Already active? (F)"=w916, "Error In"=w923, "Target VI reference"=w917) -> ("Error Out"=w919:errorcluster)  [unwired: 8 in]
    }
    frame "Image:Use ROI as Search Area" {
      # "\"Use ROI as Search Area\""
      n287 = Unbundle By Name(w933) -> ("Registered Events Ctrl Refnums.Source Image Display"=w934:refnum<vi>)
      n288 = call "AlliGator Store Search ROI.vi"("Display Image Control Refnum"=w934) -> ("Error Out"=w935:errorcluster, "Message"=w931:string)  [unwired: 8 in, 1 out]
    }
    frame "Image:Check Current ROI" {
      # "Image:Check Current ROI"
      n289 = Variant To Data(Variant=w941) -> (data=w940:T26)  [unwired: 2 in, 1 out]
      n290 = call "AlliGator Check Current Source Image ROI.vi"("Error In"=w938, "ROI Descriptor"=w940) -> ("Error Out"=w939:errorcluster)  [unwired: 7 in, 2 out]
    }
    frame "Image:Update True Pixel Value" {
      # "\"Image:Update True Pixel Value\""
      n291 = call "AlliGator Display True Pixel Value.vi"("AlliGator Ctrl Refnums"=w949, "error in (no error)"=w945, "AlliGator IV DVR in"=w947) -> ("error out"=w948:errorcluster, "AlliGator IV DVR out"=w946:refnum<data-value>)  [unwired: 7 in]
    }
  }
  "AlliGator IV DVR out" <- w18
  "error out" <- w1
  "Script out" <- w11
  "Alligator Queue Elements" <- w10
  n292 = call "Get Current Message Text Format.vi"("Text Format"=w3) -> ("Error Out"=w2:errorcluster, "Message Formatting"=w6:T2)  [unwired: 8 in]
  n293 = call "AlliGator Package Notebook Messages.vi"("Error In"=w2, "Message Formatting"=w6, "Message"=w5, "AlliGator Q Event in"="AlliGator Q Event in") -> ("[Notebook Message]"=→"[Notebook Message]":T1[])  [unwired: 6 in, 1 out]
